vi "信号光谱9-Au-卍 .vi"() -> ()   [LabVIEW 2018]
uses:
  <vilib>/Utility/NIReport.llb/Report Type.ctl
  <vilib>/Utility/file.llb/Write Delimited Spreadsheet (DBL).vi
  <vilib>/Instr/_visa.llb/VISA Configure Serial Port (Instr).vi
  <vilib>/addons/_office/excel.llb/Excel Get Data ([str]).vi
  <vilib>/Utility/NIReport.llb/NI_report.lvclass
  <vilib>/Analysis/NI_AALBase.lvlib
  <vilib>/ptbypt/NI_PtbyPt.lvlib
  <vilib>/Utility/NIReport.llb/NI_ReportGenerationCore.lvlib
  <vilib>/addons/_office/NI_ReportGenerationToolkit.lvlib
  <vilib>/Utility/NIReport.llb/Excel/NI_Excel.lvclass
panel:
  out "temp":i32
  in  "num":i32=2
  in  "角度判断下限":dbl=1.0 format="%#_13g"
  in  "角度判断上限":dbl=4.0 format="%#_13g"
  out "原始峰值":dbl
  out "拟合峰值":dbl
  in  "角度倍乘系数":dbl=1.5
  out "结果展示":dbl[][](array[numeric])=[[37.33100777239877, 2672.955043835526, 29.54153292599307, 222755.0, 50.0], [37.36593979472361, 2672.656498058864, 30.113284142729572, 222833.0, 50.0], [38.96986225690859, 2673.3337152325566, 33.38805102415213, 222910.0, 75.0], [37.39946104045098, 2676.4005085744548, 31.215565446104666, 222948.0, 47.0], [35.862209164247574, 2671.7826876859012, 30.355582265151796, 223028.0, 47.0]]
  out "Δw2>C":bool=TRUE
  out "Δw1>C":bool=TRUE
  out "θi":dbl
  in  "w0":dbl format="%#_13g"
  in  "C=w-w0":dbl=180.0 format="%#_13g"
  in  "上升下降沿/s":dbl format="%.2p"
  in  "延时/s":dbl format="%.2p"
  in  "占空比/%":dbl=3.0 format="%.2p"
  in  "高电平/V":dbl=4.0 format="%.2p"
  in  "频率/Hz":dbl=6000.0 format="%.3p"
  in  "低电平/V":dbl min=0.0 max=5.0 format="%.2p"
  in  "Enable":bool
  in  "上升下降沿":i32(ring)=1 items=["上升沿", "下降沿"]
  in  "输出信号波形":u16(ring) items=["Pulse"]
  out "Output":bool
  in  "VISA 信号发生器":refnum<visa-resource-name>="USB0::0x1AB1::0x0641::DG4E192200870::INSTR"
  out "Output 2":bool
  in  "Enable 2":bool
  in  "上升下降沿/s 2":dbl format="%.2p"
  in  "延时/s 2":dbl format="%.2p"
  in  "占空比/% 2":dbl=3.0 format="%.2p"
  in  "高电平/V 2":dbl=0.002 format="%.2p"
  in  "频率/Hz 2":dbl=6000.0 format="%.3p"
  in  "低电平/V 2":dbl min=0.0 max=5.0 format="%.2p"
  in  "上升下降沿 2":i32(ring)=1 items=["上升沿", "下降沿"]
  in  "输出信号波形 2":u16(ring) items=["Pulse"]
  in  "终止测量":bool
  in  "测量次数":i32=1
  out "best fit":cluster{"Y":dbl[], "Y":dbl[]}[](graph)
  in  "拟合终点":i32=850
  in  "拟合起点":i32=200
  out "angle":dbl
  out "图片地址":string
  in  "开光时间/ms":u32=50
  out "最终存储路径 2":path
  out "照明光error out":errorcluster
  in  "照明光":bool
  in  "stop bits (10: 1 bit)":u16(ring)=10 items=["1.0"=10, "1.5"=15, "2.0"=20]
  in  "parity (0:none)":enum16{"None", "Odd", "Even", "Mark", "Space"}(ring)
  in  "data bits (8)":u16=8 min=5 max=8 step=1
  in  "baud rate":u32=9600 caption="baud rate (115200)" min=9600 max=115200
  in  "照明光VISA":refnum<visa-resource-name>="COM6"
  out "正在测量":bool
  in  "滤波阈值":dbl=3000.0 format="%#_13g"
  out "范围内？":bool[](array[boolean])
  out "w":dbl
  out "xc":dbl
  out "拟合参数":dbl[](array[numeric])
  out "最终存储路径":path
  in  "停止程序":bool
  out "configure error out":errorcluster
  in  "设置参数":bool
  out "output control error  4":errorcluster
  in  "低电平持续输出":bool
  out "output control error  5":errorcluster
  out "output control error":errorcluster
  in  "开始测量":bool
  in  "channel输出口":i32(ring) items=["Channel 1", "Channel 2"]
  out "output control error":errorcluster
  out "Spectrum":cluster{"Y":dbl[], "Y":dbl[]}[](graph)
  out "波长范围":dbl[](array[numeric])
  in  "?":enum32{"IHR 550", "CCD"}(tab)
  in  "Move To\nTarget Positions":bool
  out "Current UniqueID":string="Mono4"
  in  "Mono ID":string(combo)="Mono1"
  in  "Connect":bool
  out "Initialized JY":bool=TRUE
  in  "Force\nInitialization":bool
  in  "Target Grating":string(combo)="2"
  out "Current Description":string="1" caption="Description"
  out "Grating Index":i32=1
  out "Current Grating":dbl=1200.0
  out "Units":string="nm"
  out "Current WL":dbl=897.9988
  out "Exit Mirror\nPosition":i32(ring)=2 items=["EntranceMirror", "ExitMirror", "Front", "Side"]
  out "Entrance Mirror\nPosition":i32(ring)=2 items=["EntranceMirror", "ExitMirror", "Front", "Side"]
  out "Units 2":string="mm"
  out "Front Entrance":dbl
  in  "Target WL":dbl=516.0
  in  "Exit Mirror":u16(ring)=3 caption="Target Position Exit Mirror" items=["Front"=2, "Side"=3]
  in  "Entrance Mirror":u16(ring)=2 caption="Target Position\nEntrance Mirror" items=["Front"=2, "Side"=3]
  in  "Target\nFront Entrance":dbl=2.0
  in  "Commande tab":T1(tab)
  in  "Area Number to Display":i32
  in  "Reformat":bool
  in  "GAIN":u16(ring)=2 caption="Device Name" items=["High Light", "Best Dynamic Range", "High Sensitivity"]
  in  "ADC":u16(ring) caption="Device Name" items=["20 kHz       ", " 1 MHz       ", " 1 MHz Ultra "]
  in  "Number of Areas :":u16=1 min=1 step=1
  in  "Integration time (ms) :":i16=1000
  out "Uniques ID":u16(ring) items=["CCD1", "CCD2"]
  in  "Device Name":u16(ring) items=["Synapse CCD (Lateral)", "Synapse_IGA (Axial)"]
  in  "Signal type :":enum16{"TTL Rising Edge", "TTL Falling Edge"}(ring)=enum."TTL Falling Edge"
  in  "Trigger Type :":u16(ring) items=["On Start"=1, "Per Acquisition"=2]
  in  "trigSigTypeString":string
  in  "trigEventString":string
  in  "Enable InputTriggers :":bool
  in  "Number of Cleans":i32=1
  in  "MultiAcqShutterMode":i32(ring)=3 items=["Open For All Spectra"=1, "Open for Each Spectrum"=3]
  in  "Accumulations:":u16=10 min=1 step=1
  in  "Multi Accumulation mode:":bool
  out "Y Pixels:":i32=256
  out "DataSize":i32=1024
  out "X Pixels:":i32=1024
  out "Firmware\nVersion":string="V1.20 CCD_4000"
  out "initialized ?":bool=TRUE
  in  "Continuous":bool
  in  "CCD Busy":bool
  out "indicator":string="Ready !"
  in  "initialize":bool
  in  "ShutterOpen":bool=TRUE caption="Shutter enable"
  in  "Acquire":bool
  in  "Temperature":bool
  in  "Setup":bool
  out "Acq Time(ms)":u32=3401
  in  "Save Backlight":bool
  in  "cut backlight":bool
  out "backlight":bool=TRUE
  in  "是否拟合":bool
  in  "是否保存":bool
  in  "Close":bool=TRUE
  out "JYCCDLib.IJYCCDReqd":refnum<k7>
  out "areas :":i32[][](array[numeric])=[[1], [1], [1], [1024], [256], [1], [256]]
  in  "Constante de condition\n(Voir l'aide contextuelle)":bool
  out "temp graph":dbl(graph)=-134.538067
  out "ADC Number":i32[](array[numeric])=[0, 1, 2, 3, 4]
  out "Gain Number":i32[](array[numeric])=[10, 11, 12, 13, 8, 2]
  out "trigAddress":i32
  out "Data":i32[][](graph)
  out "error out":errorcluster
  out "Gratings":dbl[](array[numeric])=[1200.0, 300.0]
  out "Backlight":i32[][](graph)
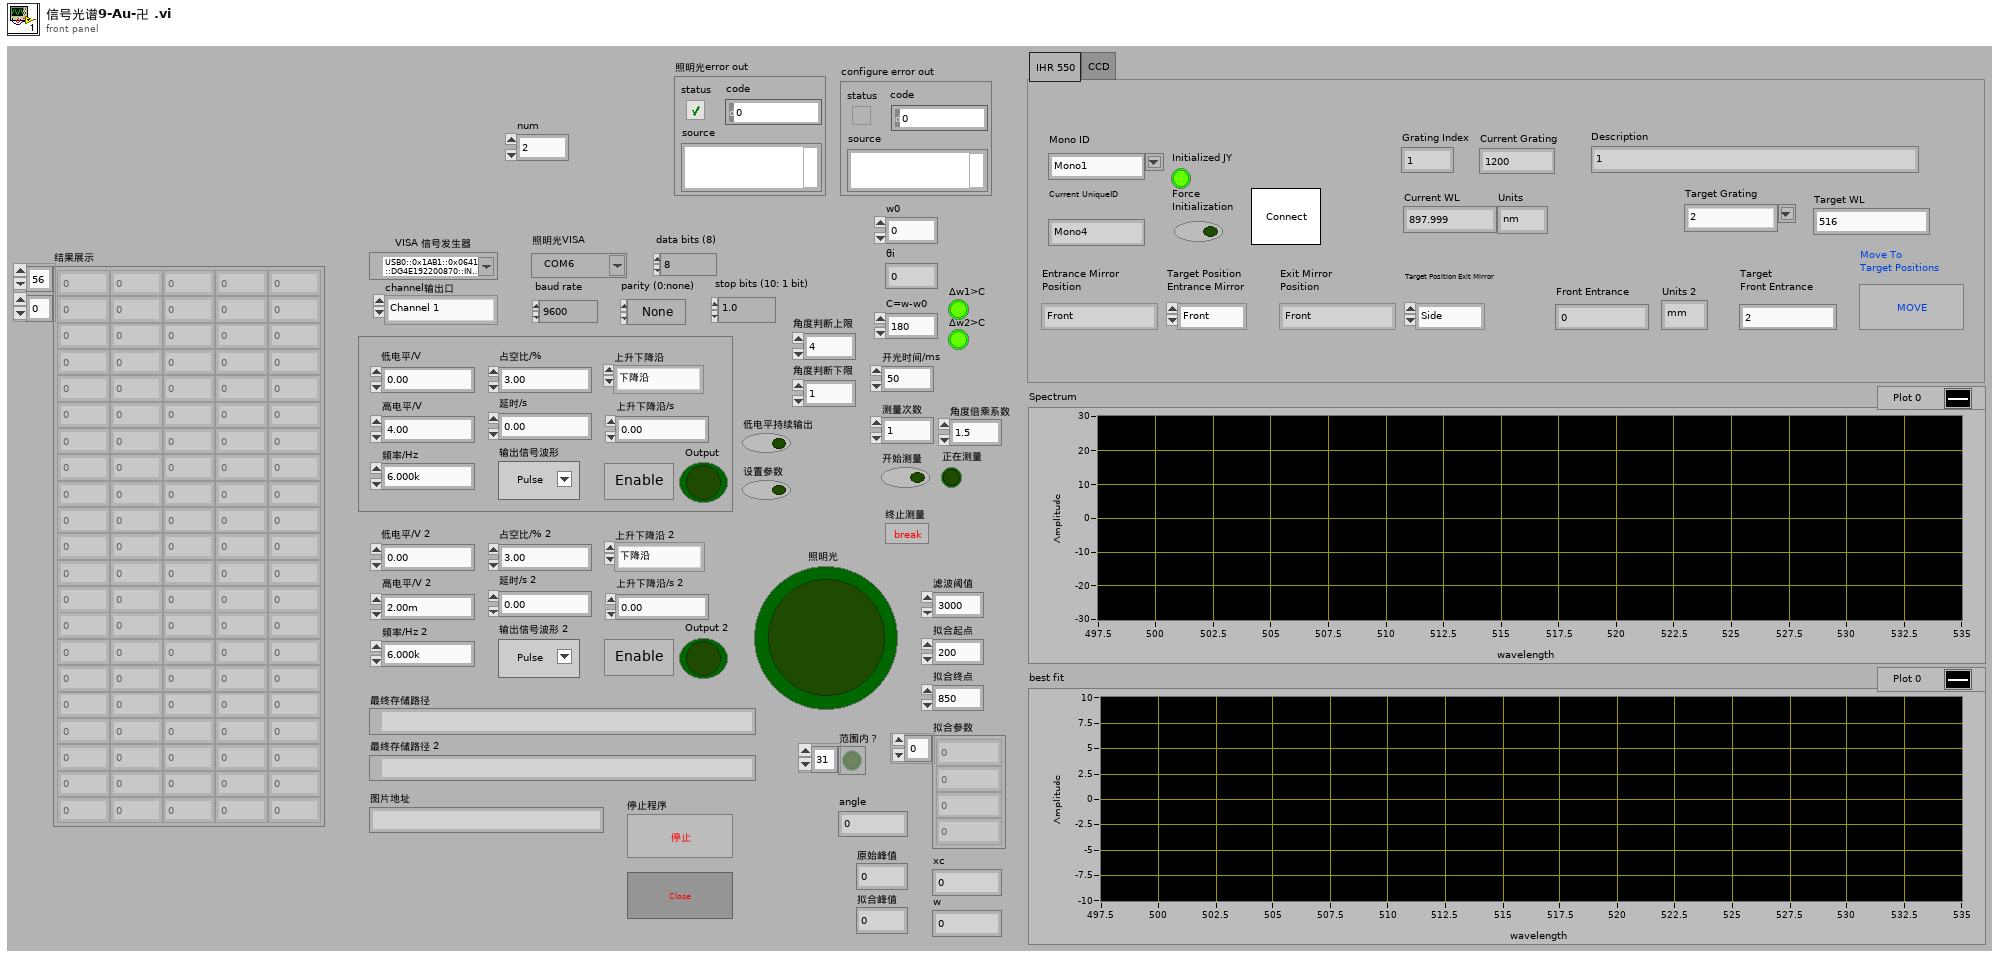
[diagram p1: front panel]
types:
  T1 = enum32{"Settings", "Trigger In", "Multi-Accu.", "Infos"}
  T2 = enum8{"Enabled", "Disabled", "Disabled and Grayed Out"}
  T3 = enum16{"maximized", "minimized", "normal", "no change"}
  T4 = typedef "NI_ReportGenerationCore.lvlib/Report Type.ctl" = enum16{"HTML", "Word", "Excel"}
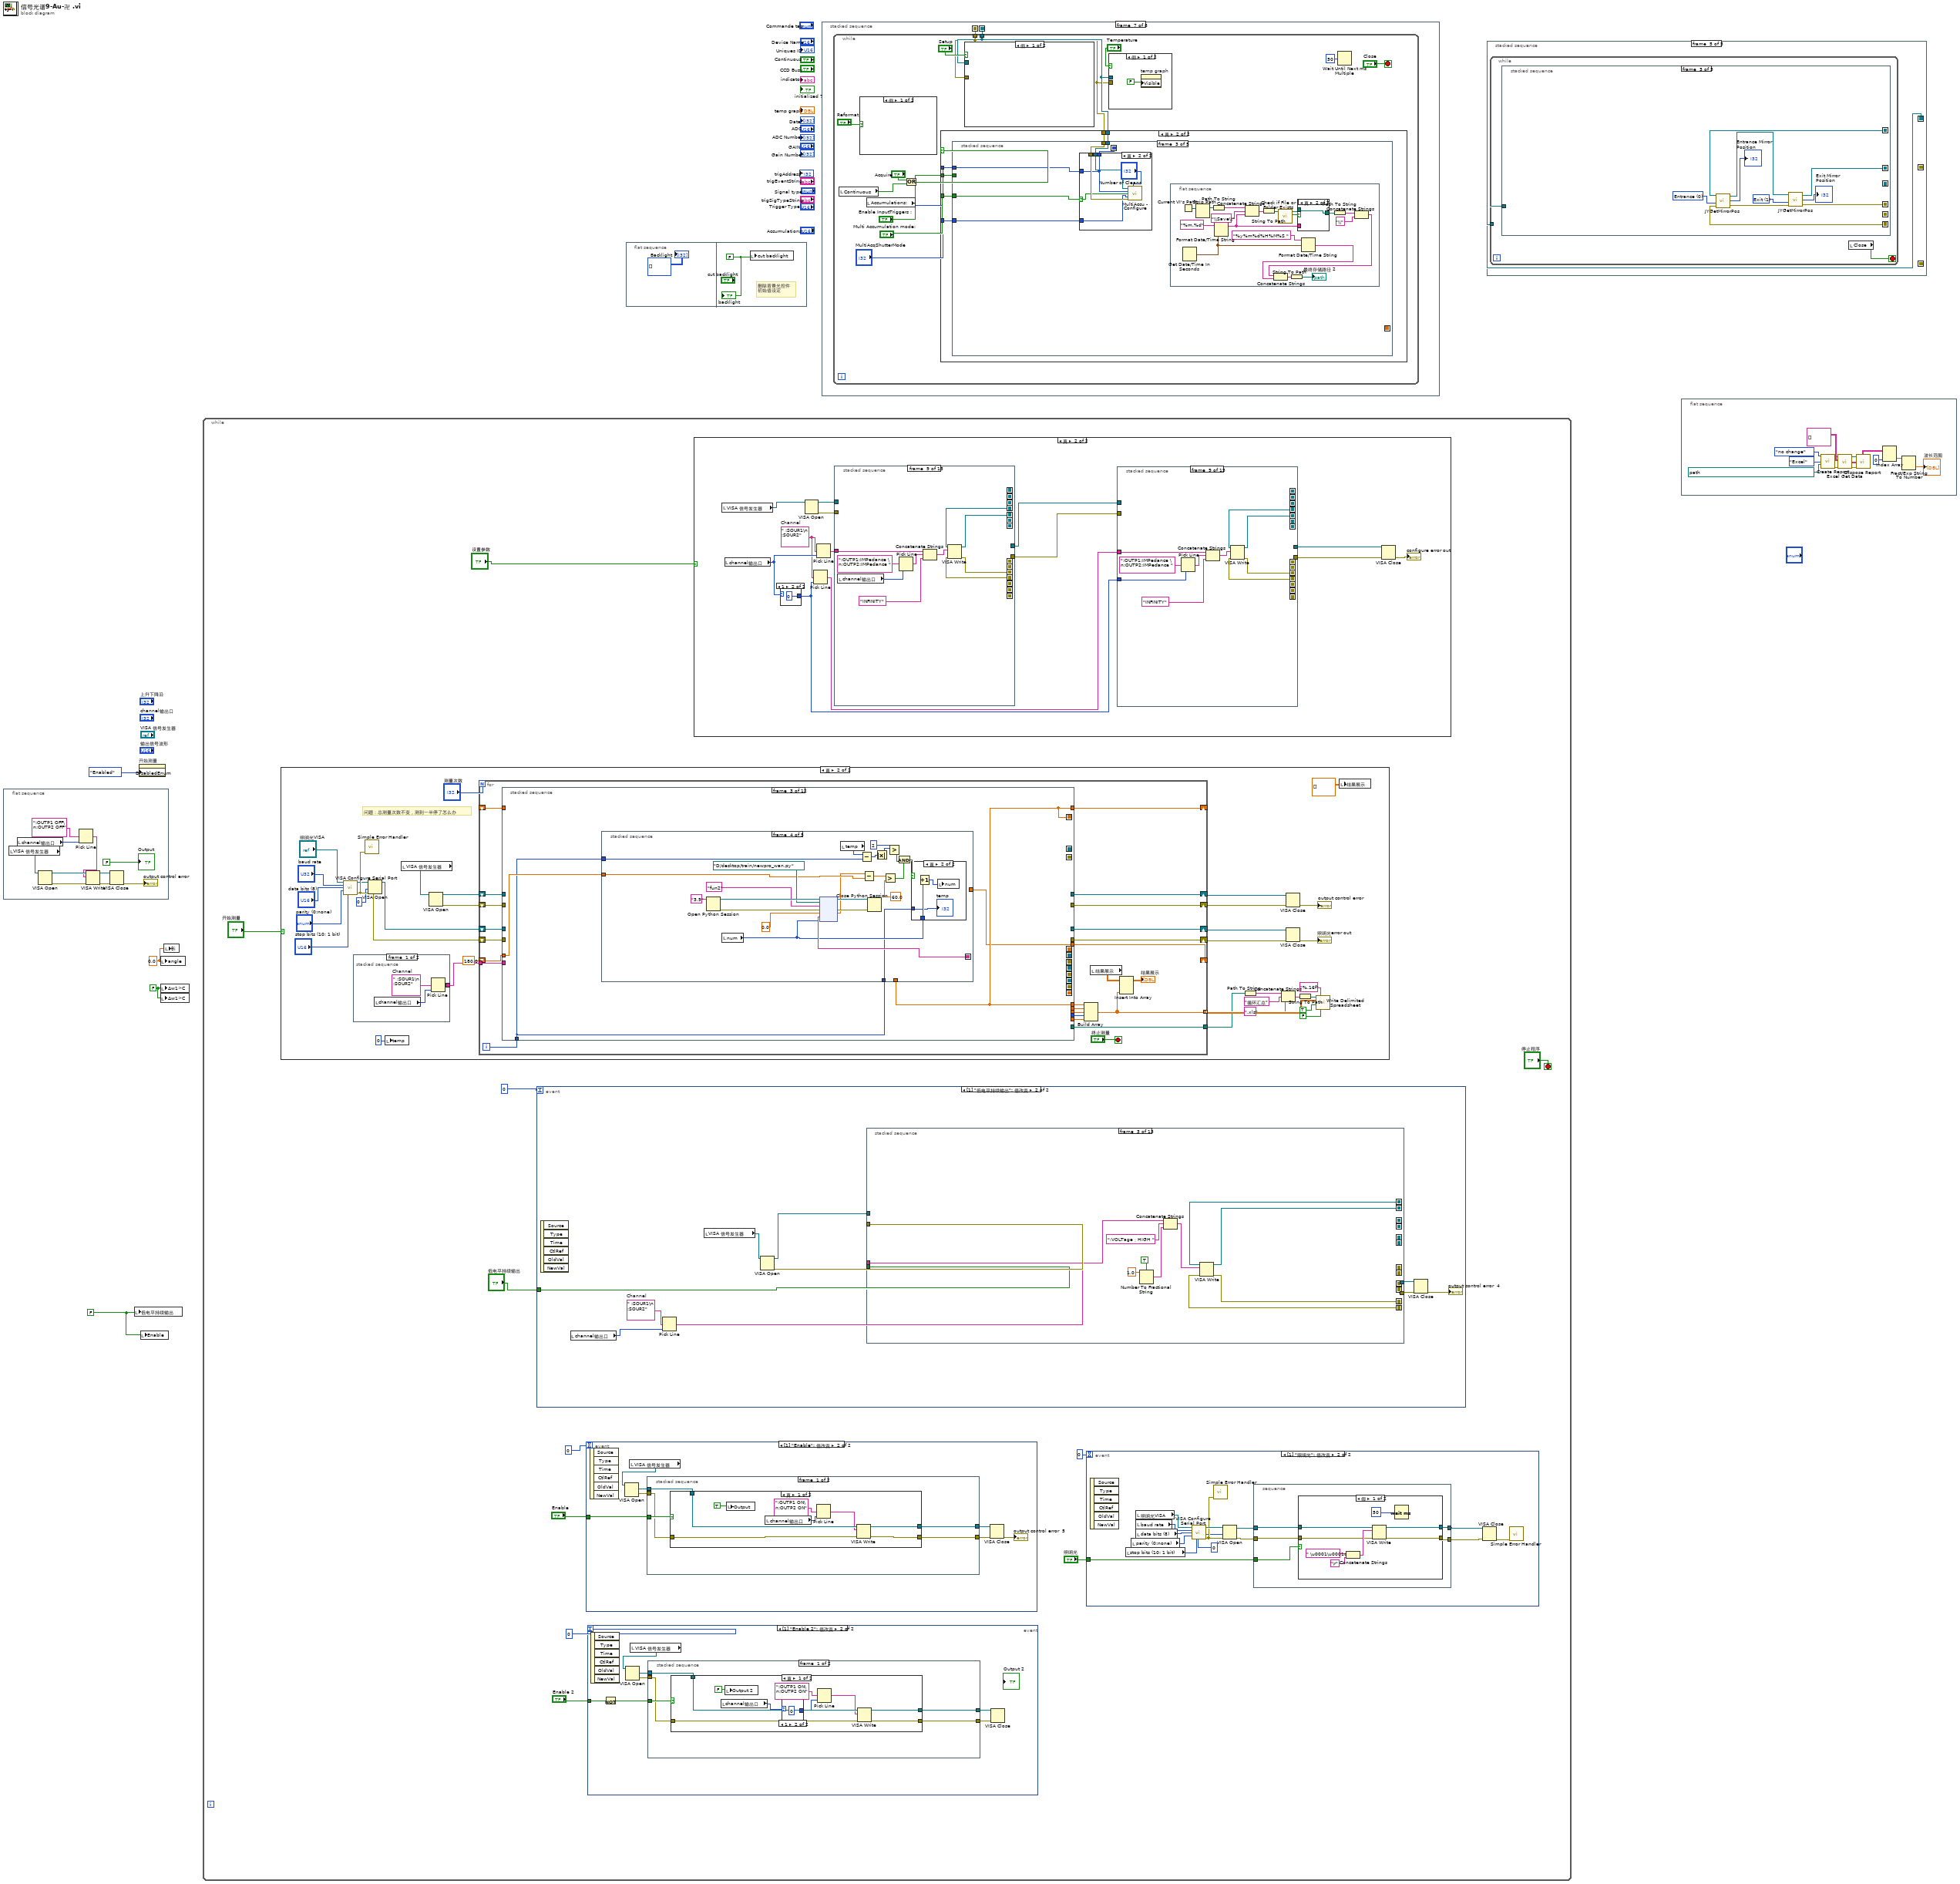
[diagram p0: block diagram]
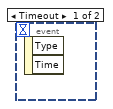
[diagram p2: hidden frame]
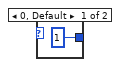
[diagram p3: hidden frame]
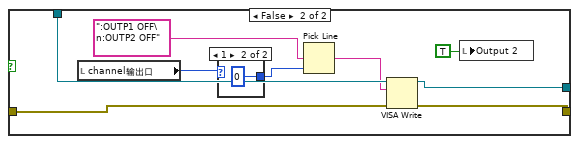
[diagram p4: hidden frame]
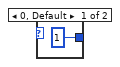
[diagram p5: hidden frame]
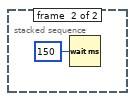
[diagram p6: hidden frame]
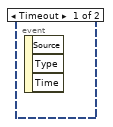
[diagram p7: hidden frame]
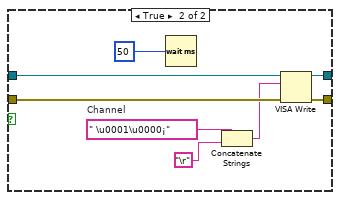
[diagram p8: hidden frame]
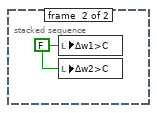
[diagram p10: hidden frame]
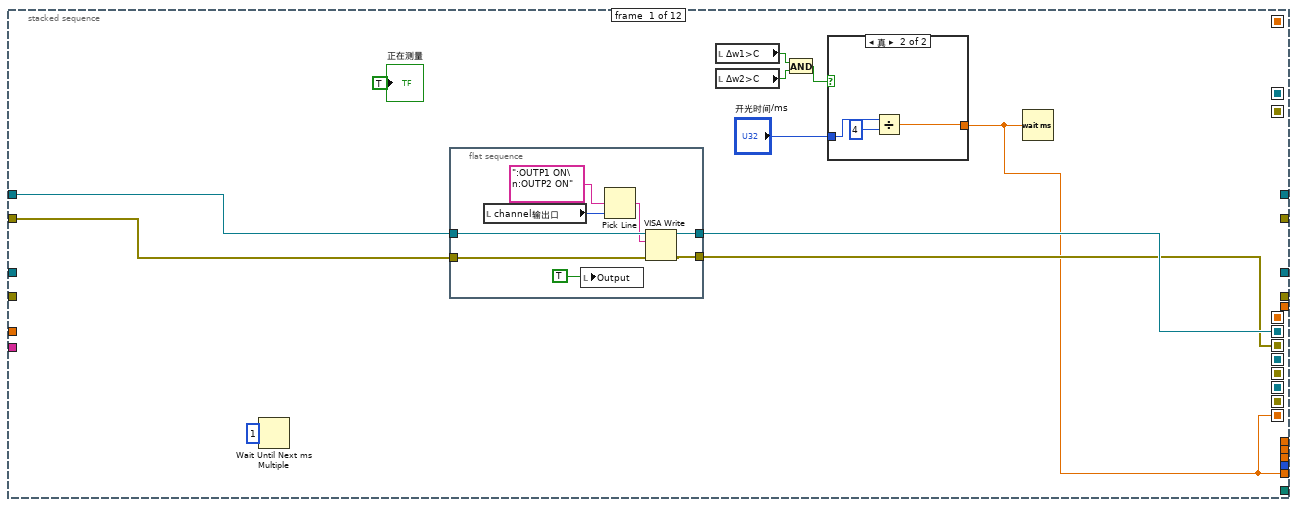
[diagram p11: hidden frame]
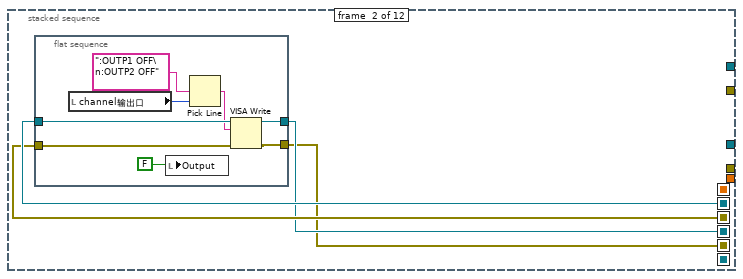
[diagram p13: hidden frame]
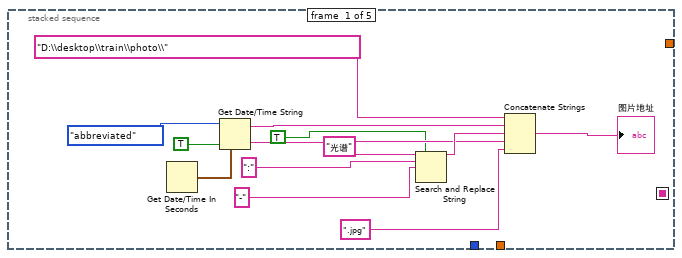
[diagram p14: hidden frame]
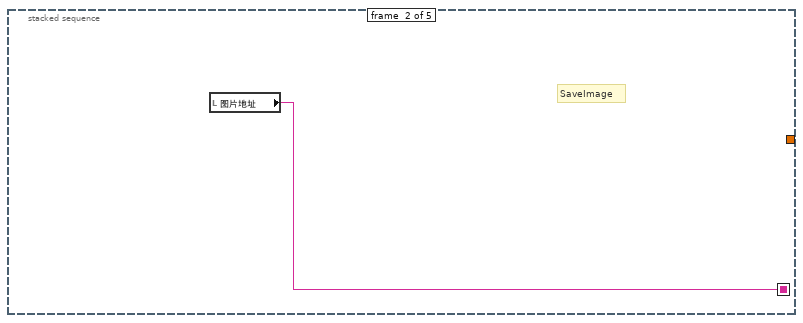
[diagram p15: hidden frame]
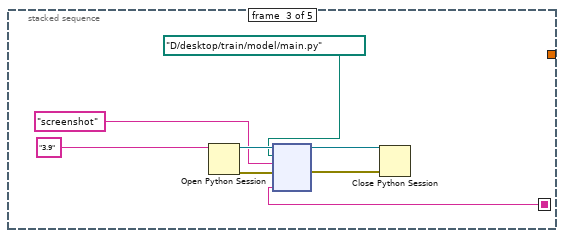
[diagram p16: hidden frame]
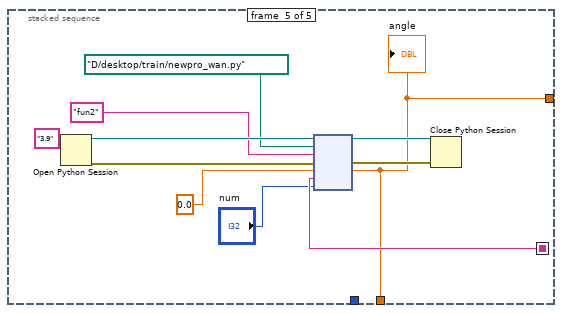
[diagram p18: hidden frame]
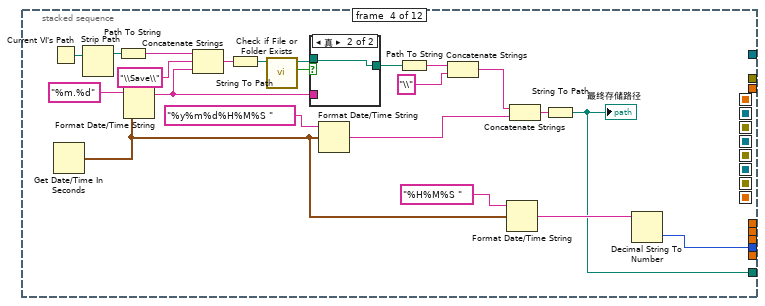
[diagram p19: hidden frame]
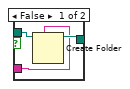
[diagram p20: hidden frame]
diagram:
  w1 = FALSE ("Δw1>C")
  w2 = 0.0 ("angle")
  w3 = FALSE
  n1 = flat-sequence {
    frame #0 {
      n2 = local read "VISA 信号发生器"() -> (w8:refnum<visa-resource-name>)
      n3 = local read "channel输出口"() -> (w6:i32)
      n4 = VISA Open(VISA resource name=w8) -> (VISA resource name=w14:refnum<visa-resource-name>, error out=w13:errorcluster)  [unwired: 4 in]
      n5 = Pick Line(multi-line string=":OUTP1 OFF\n:OUTP2 OFF" ("write buffer"), line index=w6) -> (output string=w5:string)  [unwired: 1 in]
      n6 = VISA Write(VISA resource name=w14, write buffer=w5, error in (no error)=w13) -> (VISA resource name out=w11:refnum<visa-resource-name>, error out=w10:errorcluster)  [unwired: 1 out]
      n7 = VISA Close(VISA resource name=w11, error in (no error)=w10) -> (error out=→"output control error":errorcluster)
      "Output" <- FALSE ("布尔")
    }
  }
  n8 = local write "低电平持续输出"(w3) -> ()
  n9 = property on="开始测量" class="Bool"("DisabledEnum"=T2."Enabled" ("禁用")) -> ()  [unwired: 2 in, 2 out]
  n10 = local write "Enable"(w3) -> ()
  n11 = local write "angle"(w2) -> ()
  n12 = local write "Δw1>C"(w1) -> ()
  n13 = local write "Δw1>C"(w1) -> ()
  n14 = local write "θi"(w2) -> ()
  n15 = while {
    stop <- "停止程序" stop-if-true
    n16 = case shown="真" "开始测量" {
      frame False {
      }
      frame True {
        # "问题：总测量次数不变，测到一半停了怎么办"
        n17 = call-poly "VISA Configure Serial Port"("VISA resource name"="照明光VISA", "baud rate (9600)"="baud rate", "data bits (8)"="data bits (8)", "parity (0:none)"="parity (0:none)", "stop bits (10: 1 bit)"="stop bits (10: 1 bit)") -> ("VISA resource name out"=w120:refnum<visa-resource-name>, "error out"=w121:errorcluster)  [unwired: 9 in]
        n18 = stacked-sequence {
          tunnel: [w130 _] -> w124
          frame #0 {
            w131 = " :SOUR1\n :SOUR2"  # Channel
            n19 = local read "channel输出口"() -> (w132:i32)
            n20 = Pick Line(multi-line string=w131, line index=w132) -> (output string=w130:string)  [unwired: 1 in]
          }
          frame #1 {
            w133 = FALSE ("Δw1>C")
            n21 = local write "Δw1>C"(w133) -> ()
            n22 = local write "Δw2>C"(w133) -> ()
          }
        }
        n23 = call <vilib>:"Simple Error Handler.vi"("error in (no error)"=w121) -> ()  [unwired: 4 in, 5 out]
        n24 = VISA Open(access mode=0, error in (no error)=w121, VISA resource name=w120) -> (VISA resource name=w113:refnum<visa-resource-name>, error out=w112:errorcluster)  [unwired: 2 in]
        n25 = local write "temp"(0 ("temp")) -> ()
        n26 = local read "VISA 信号发生器"() -> (w129:refnum<visa-resource-name>)
        n27 = VISA Open(VISA resource name=w129) -> (VISA resource name=w128:refnum<visa-resource-name>, error out=w127:errorcluster)  [unwired: 4 in]
        n28 = for {
          N: "测量次数" -> [_]
          tunnel: w124 -> [w155]
          shift-right: [w151] -> w123
          shift-left: w128 -> [w157]
          shift-right: [w150] -> w122
          shift-left: w127 -> [w156]
          shift-right: [w149] -> w126
          shift-left: w113 -> [w154]
          shift-right: [w148] -> w125
          shift-left: w112 -> [w153]
          tunnel: [w138] -> w102 mode=indexing
          shift-right: [w143] -> _
          shift-left: _ -> [w142]
          tunnel: [w139] -> w99
          shift-right: [w135] -> _
          shift-left: 180.0 -> [w134]
          i -> [w141]
          stop <- "终止测量" stop-if-true
          n29 = stacked-sequence {
            seq-local: [w164 _ _ _ _ _ _ _ _ _ _ _] -> [_ w184 _ _ _ _ _ _ _ _ _ _]
            seq-local: [w163 _ _ _ _ _ _ _ _ _ _ _] -> [_ w183 _ _ _ _ _ _ _ _ _ _]
            seq-local: [_ _ _ _ _ w299 _ _ _ _ _ _] -> [_ _ _ _ _ _ _ _ w417 _ _ _]
            seq-local: [_ _ _ _ _ w298 _ _ _ _ _ _] -> [_ _ _ _ _ _ _ _ w420 _ _ _]
            seq-local: [_ w182 _ _ _ _ _ _ _ _ _ _] -> [_ _ _ _ w285 _ _ _ _ _ _ _]
            seq-local: [_ w181 _ _ _ _ _ _ _ _ _ _] -> [_ _ _ _ w284 _ _ _ _ _ _ _]
            seq-local: [_ _ _ _ w283 _ _ _ _ _ _ _] -> [_ _ _ _ _ _ _ w403 _ _ _ _]
            seq-local: [_ _ _ _ w282 _ _ _ _ _ _ _] -> [_ _ _ _ _ _ _ w402 _ _ _ _]
            seq-local: [_ _ w196 _ _ _ _ _ _ _ _ _] -> [_ _ _ _ _ _ _ _ _ _ w429 _]
            seq-local: [_ _ _ _ _ _ w312 _ _ _ _ _] -> [_ _ _ _ _ _ _ _ _ _ w424 _]
            seq-local: [w158 _ _ _ _ _ _ _ _ _ _ _] -> [_ _ _ _ _ _ w310 _ _ _ _ _]
            tunnel: w157 -> [w166 _ _ _ _ _ _ _ _ _ _ _]
            tunnel: w156 -> [w165 _ _ _ _ _ _ _ _ _ _ _]
            tunnel: [_ _ _ _ _ _ _ w401 _ _ _ _] -> w151
            tunnel: [_ _ _ _ _ _ _ w400 _ _ _ _] -> w150
            tunnel: w155 -> [_ _ _ _ _ _ _ _ _ _ _ _]
            tunnel: w154 -> [_ _ _ _ _ w302 _ _ _ _ _ _]
            tunnel: w153 -> [_ _ _ _ _ w301 _ _ _ _ _ _]
            tunnel: [_ _ _ _ _ _ _ _ w419 _ _ _] -> w149
            tunnel: [_ _ _ _ _ _ _ _ w418 _ _ _] -> w148
            tunnel: [_ _ w196 _ _ _ _ _ _ _ _ _] -> w147
            tunnel: [_ _ _ _ _ _ w307 _ _ _ _ _] -> w146
            tunnel: [_ _ _ _ _ _ w306 _ _ _ _ _] -> w145
            tunnel: [_ _ _ w257 _ _ _ _ _ _ _ _] -> w144
            tunnel: [w158 _ _ _ _ _ _ _ _ _ _ _] -> w140
            tunnel: [_ _ w196 _ _ _ _ _ _ _ _ _] -> w143
            tunnel: w142 -> [_ _ _ _ _ _ _ _ _ _ w428 _]
            tunnel: w141 -> [_ _ w193 _ _ _ _ _ _ _ w426 _]
            tunnel: [_ _ _ w256 _ _ _ _ _ _ _ _] -> w139
            tunnel: [_ _ w195 _ _ _ _ _ _ _ _ _] -> w135
            tunnel: w134 -> [_ _ w194 _ _ _ _ _ _ _ _ _]
            frame #0 {
              n30 = Wait Until Next ms Multiple(millisecond multiple=u32 1 ("毫秒倍数")) -> ()  [unwired: 1 out]
              n31 = flat-sequence {
                tunnel: w166 -> [w180]
                tunnel: w165 -> [w179]
                tunnel: [w174] -> w164
                tunnel: [w173] -> w163
                frame #0 {
                  n32 = local read "channel输出口"() -> (w176:i32)
                  n33 = local write "Output"(TRUE ("布尔")) -> ()
                  n34 = Pick Line(multi-line string=":OUTP1 ON\n:OUTP2 ON" ("write buffer"), line index=w176) -> (output string=w175:string)  [unwired: 1 in]
                  n35 = VISA Write(VISA resource name=w180, write buffer=w175, error in (no error)=w179) -> (VISA resource name out=w174:refnum<visa-resource-name>, error out=w173:errorcluster)  [unwired: 1 out]
                }
              }
              n36 = local read "Δw1>C"() -> (w160:bool)
              n37 = local read "Δw2>C"() -> (w161:bool)
              n38 = And(x=w160, y=w161) -> (x .and. y?=w159:bool)
              n39 = case shown="真" w159 {
                tunnel: [w169 w170] -> w158
                tunnel: "开光时间/ms" -> [w169 w172]
                frame False {
                }
                frame True {
                  n40 = Divide(x=w172, y=u32 4) -> (x/y=w170:dbl)
                }
              }
              n41 = Wait (ms)(milliseconds to wait=w158) -> ()  [unwired: 1 out]
              "正在测量" <- TRUE
            }
            frame #1 {
              n42 = flat-sequence {
                tunnel: w184 -> [w192]
                tunnel: w183 -> [w191]
                tunnel: [w186] -> w182
                tunnel: [w185] -> w181
                frame #0 {
                  n43 = local read "channel输出口"() -> (w188:i32)
                  n44 = local write "Output"(FALSE ("布尔")) -> ()
                  n45 = Pick Line(multi-line string=":OUTP1 OFF\n:OUTP2 OFF" ("write buffer"), line index=w188) -> (output string=w187:string)  [unwired: 1 in]
                  n46 = VISA Write(VISA resource name=w192, write buffer=w187, error in (no error)=w191) -> (VISA resource name out=w186:refnum<visa-resource-name>, error out=w185:errorcluster)  [unwired: 1 out]
                }
              }
            }
            frame #2 {
              n47 = stacked-sequence {
                seq-local: [_ w210 _ _ _] -> [_ _ w211 w233 w247]
                tunnel: [_ _ _ _ w245] -> w196
                tunnel: [_ _ _ _ w245] -> w195
                tunnel: w194 -> [_ _ _ w229 _]
                tunnel: w193 -> [_ _ _ w225 _]
                tunnel: w193 -> [_ _ _ w223 _]
                frame #0 {
                  n48 = Get Date/Time In Seconds() -> (seconds since 1Jan1904=w206:timestamp)
                  n49 = Get Date/Time String(date format (0)=enum16{"short", "long", "abbreviated"}."abbreviated" ("日期格式(0)"), seconds (now)=w206, want seconds? (F)=TRUE ("需要秒？(F)")) -> (date string=w209:string, time string=w207:string)
                  n50 = Search and Replace String(replace all?=TRUE ("替换全部？(F)"), input string=w207, search string=":" ("搜索字符串"), replace string="-" ("替换字符串(\"\")")) -> (result string=w208:string)  [unwired: 4 in, 3 out]
                  n51 = Concatenate Strings("D:\\desktop\\train\\photo\\", w209, w208, "光谱" ("字符串"), ".jpg" ("字符串")) -> (→"图片地址":string)
                }
                frame #1 {
                  # "SaveImage"
                  n52 = local read "图片地址"() -> (w210:string)
                }
                frame #2 {
                  n53 = Open Python Session(python version="3.9" ("Python version")) -> (session out=w218:refnum<k35>, error out=w216:errorcluster)  [unwired: 2 in]
                  n54 = node(w218, path "D:/desktop/train/model/main.py" ("module path"), "screenshot" ("function name"), w216, w211) -> (w217:refnum<k35>, w215:errorcluster)  [unwired: 3 in, 2 out]
                  n55 = Close Python Session(session in=w217, error in=w215) -> ()  [unwired: 1 out]
                }
                frame #3 {
                  n56 = Open Python Session(python version="3.9" ("Python version")) -> (session out=w240:refnum<k35>, error out=w238:errorcluster)  [unwired: 2 in]
                  n57 = local read "num"() -> (w230:i32)
                  n58 = node(w240, path "D:/desktop/train/newpro_wan.py" ("module path"), "fun2" ("function name"), w238, 0.0, w233, w230) -> (w239:refnum<k35>, w237:errorcluster, w228:dbl)  [unwired: 2 in, 2 out]
                  n59 = local read "temp"() -> (w224:i32)
                  n60 = Subtract(x=w224, y=w223) -> (x-y=w222:i32)
                  n61 = Subtract(x=w228, y=w229) -> (x-y=w232:dbl)
                  n62 = Close Python Session(session in=w239, error in=w237) -> ()  [unwired: 1 out]
                  n63 = Absolute Value(x=w222) -> (abs(x)=w221:i32)
                  n64 = Greater?(x=w232, y=60.0) -> (0:w227:bool)
                  n65 = Greater?(x=w221, y=2) -> (0:w220:bool)
                  n66 = And(x=w227, y=w220) -> (x .and. y?=w226:bool)
                  n67 = case shown="真" w226 {
                    tunnel: w230 -> [_ w244]
                    tunnel: w225 -> [_ w242]
                    frame False {
                    }
                    frame True {
                      n68 = Increment(x=w244) -> (x+1=w243:i32)
                      n69 = local write "num"(w243) -> ()
                      "temp" <- w242
                    }
                  }
                }
                frame #4 {
                  n70 = Open Python Session(python version="3.9" ("Python version")) -> (session out=w254:refnum<k35>, error out=w252:errorcluster)  [unwired: 2 in]
                  n71 = node(w254, path "D:/desktop/train/newpro_wan.py" ("module path"), "fun2" ("function name"), w252, 0.0, w247, "num") -> (w253:refnum<k35>, w251:errorcluster, w245:dbl)  [unwired: 2 in, 2 out]
                  "angle" <- w245
                  n72 = Close Python Session(session in=w253, error in=w251) -> ()  [unwired: 1 out]
                }
              }
            }
            frame #3 {
              n73 = Current VI's Path() -> (path=w266:path)
              n74 = Get Date/Time In Seconds() -> (seconds since 1Jan1904=w259:timestamp)
              n75 = Strip Path(path=w266) -> (stripped path=w267:path)  [unwired: 1 out]
              n76 = Path To String(path=w267) -> (string=w268:string)
              n77 = Format Date/Time String(time format string (%c)="%m.%d" ("时间格式字符串(%c)"), seconds (now)=w259) -> (date/time string=w274:string)  [unwired: 1 in]
              n78 = Concatenate Strings(w268, "\\Save\\" ("字符串"), w274) -> (w269:string)
              n79 = String To Path(string=w269) -> (path=w270:path)
              n80 = call <vilib>:"Check if File or Folder Exists.vi"("path"=w270) -> ("file or folder exists?"=w271:bool, "dup path"=w273:path)  [unwired: 8 in, 1 out]
              n81 = case shown="真" w271 {
                tunnel: [w280 w281] -> w272
                tunnel: w273 -> [w279 w281]
                tunnel: w274 -> [w278 _]
                frame False {
                  n82 = Create Folder(prompt (Create Folder)=w278, path (use dialog)=w279) -> (created path=w280:path)  [unwired: 1 in, 2 out]
                }
                frame True {
                }
              }
              n83 = Format Date/Time String(time format string (%c)="%y%m%d%H%M%S " ("时间格式字符串(%c)"), seconds (now)=w259) -> (date/time string=w277:string)  [unwired: 1 in]
              n84 = Path To String(path=w272) -> (string=w275:string)
              n85 = Concatenate Strings(w275, "\\" ("字符串")) -> (w276:string)
              n86 = Format Date/Time String(time format string (%c)="%H%M%S " ("时间格式字符串(%c)"), seconds (now)=w259) -> (date/time string=w258:string)  [unwired: 1 in]
              n87 = Concatenate Strings(w276, w277) -> (w265:string)
              n88 = String To Path(string=w265) -> (path=w256:path)
              "最终存储路径" <- w256
              n89 = Decimal String To Number(string=w258) -> (number=w257:i32)  [unwired: 2 in, 1 out]
            }
            frame #4 {
              n90 = flat-sequence {
                tunnel: w285 -> [w294]
                tunnel: w284 -> [w293]
                tunnel: [w289] -> w283
                tunnel: [w288] -> w282
                frame #0 {
                  n91 = local read "channel输出口"() -> (w287:i32)
                  n92 = case shown="1" w287 {
                    tunnel: [1 0] -> w286
                    frame 0, Default {
                    }
                    frame 1 {
                    }
                  }
                  n93 = local write "Output 2"(FALSE ("布尔")) -> ()
                  n94 = Pick Line(multi-line string=":OUTP1 OFF\n:OUTP2 OFF" ("write buffer"), line index=w286) -> (output string=w290:string)  [unwired: 1 in]
                  n95 = VISA Write(VISA resource name=w294, write buffer=w290, error in (no error)=w293) -> (VISA resource name out=w289:refnum<visa-resource-name>, error out=w288:errorcluster)  [unwired: 1 out]
                }
              }
            }
            frame #5 {
              w297 = " \u0001\u0001¢"  # Channel
              n96 = Wait (ms)(milliseconds to wait=1200) -> ()  [unwired: 1 out]
              n97 = Concatenate Strings(w297, "\r") -> (w303:string)
              n98 = local write "照明光"(FALSE ("照明光")) -> ()
              n99 = VISA Write(VISA resource name=w302, write buffer=w303, error in (no error)=w301) -> (VISA resource name out=w299:refnum<visa-resource-name>, error out=w298:errorcluster)  [unwired: 1 out]
            }
            frame #6 {
              n100 = local read "Area Number to Display"() -> (w353:i32)
              n101 = local read "JYCCDLib.IJYCCDReqd"() -> (w349:refnum<k7>)
              n102 = Get Date/Time In Seconds() -> (seconds since 1Jan1904=w362:timestamp)
              n103 = local read "最终存储路径"() -> (w376:path)
              n104 = Get Date/Time String(date format (0)=enum16{"short", "long", "abbreviated"}."abbreviated" ("日期格式(0)"), seconds (now)=w362, want seconds? (F)=TRUE ("需要秒？(F)")) -> (date string=w370:string, time string=w365:string)
              n105 = call "MultiAccu - Acquire spectral.vi"("error in"=errorcluster {"status"=FALSE, "code"=0, "source"=""}, "Accumulations:"=u16 1, "ShutterOpen"=TRUE, "JYCCDLib.IJYCCDReqd"=w349) -> ("Acq Time(ms)"=w355:u32, "Array Out"=w354:i32[][][])  [unwired: 1 out]
              n106 = local write "Acq Time(ms)"(w355) -> ()
              n107 = local read "cut backlight"() -> (w337:bool)
              n108 = local read "backlight"() -> (w335:bool)
              n109 = Search and Replace String(replace all?=TRUE ("替换全部？(F)"), input string=w365, search string=":" ("搜索字符串"), replace string="-" ("替换字符串(\"\")")) -> (result string=w369:string)  [unwired: 4 in, 3 out]
              n110 = Path To String(path=w376) -> (string=w359:string)
              n111 = And(x=w337, y=w335) -> (x .and. y?=w336:bool)
              n112 = call "Array reset dimension.vi"("Area Number"=w353, "Array In"=w354) -> ("Array Out"=w339:i32[][])
              n113 = Concatenate Strings(w359, w370, w369, "光谱" ("字符串"), ".xls" ("字符串")) -> (w374:string)
              n114 = case shown="真" w336 {
                tunnel: [w396 w398] -> w338
                tunnel: w339 -> [w396 w397]
                frame False {
                }
                frame True {
                  n115 = local read "Backlight"() -> (w399:i32[][])
                  n116 = Subtract(x=w397, y=w399) -> (x-y=w398:i32[][])
                }
              }
              n117 = String To Path(string=w374) -> (path=w375:path)
              n118 = local write "Data"(w339) -> ()
              n119 = local read "波长范围"() -> (w318:dbl[])
              n120 = Index Array(array=w338, index (row)=0 ("索引 (行)")) -> (element=w377:i32[])  [unwired: 1 in]
              n121 = Reverse 1D Array(array=w377) -> (reversed array=w315:i32[])
              n122 = local read "angle"() -> (w317:dbl)
              n123 = local read "拟合起点"() -> (w325:i32)
              n124 = local read "拟合终点"() -> (w327:i32)
              n125 = call <vilib>:"Median Filter.vi"("left rank"=6, "X"=w315) -> ("Filtered X"=w314:dbl[])  [unwired: 8 in, 1 out]
              n126 = Build Array(w317, w310, 0.0 ("元素")) -> (w316:dbl[])
              n127 = Subtract(x=w327, y=w325) -> (x-y=w324:i32)
              n128 = call "Convert to Dynamic Data"("Array"=w318) -> ("Dynamic Data Type"=w346:dynamicdata)  [unwired: 3 in]
              n129 = call "Convert to Dynamic Data2"("Array"=w315) -> ("Dynamic Data Type"=w345:dynamicdata)  [unwired: 3 in]
              n130 = Array Subset(array=w318, index=w325, length=w324) -> (w323:dbl[])
              n131 = call "Build XY Graph"("Y Input"=w345, "X Input"=w346) -> ("XY Graph"=→"Spectrum":cluster{"Y":dbl[], "Y":dbl[]}[])  [unwired: 8 in, 1 out]
              n132 = call "转换至动态数据4"("Array"=w323) -> ("Dynamic Data Type"=w343:dynamicdata)  [unwired: 3 in]
              n133 = In Range and Coerce(upper limit="滤波阈值", x=w314, lower limit=-100.0) -> (In Range?=w330:bool[])  [unwired: 1 out]
              "范围内？" <- w330
              n134 = Not(x=w330) -> (.not. x?=w329:bool[])
              n135 = Or Array Elements(Boolean array=w329) -> (logical OR=w332:bool)
              n136 = local read "X Pixels:"() -> (w331:i32)
              n137 = local read "波长范围"() -> (w319:dbl[])
              n138 = local read "滤波阈值"() -> (w328:dbl)
              n139 = case shown="真" w332 {
                tunnel: w331 -> [_ w383]
                tunnel: w314 -> [w379 w382]
                tunnel: [w379 w381] -> w308
                tunnel: w328 -> [_ w380]
                frame False {
                }
                frame True {
                  n140 = for {
                    N: w383 -> [_]
                    tunnel: w382 -> [w387] mode=indexing
                    tunnel: [w386] -> w381 mode=indexing
                    shift-right: [w386] -> _
                    shift-left: _ -> [w385]
                    tunnel: w380 -> [w384]
                    n141 = Greater?(x=w387, y=w384) -> (0:w389:bool)
                    n142 = Less?(x=w387, y=-100.0) -> (x < y?=w390:bool)
                    n143 = Or(x=w389, y=w390) -> (x .or. y?=w388:bool)
                    n144 = case shown="真" w388 {
                      tunnel: w387 -> [w392 _]
                      tunnel: [w392 w394] -> w386
                      tunnel: w385 -> [_ w395]
                      frame False {
                      }
                      frame True {
                        n145 = call <vilib>:"Median Filter PtByPt.vi"("rank"=5, "x"=w395) -> ("Filtered x"=w394:dbl)  [unwired: 2 in, 1 out]
                      }
                    }
                  }
                }
              }
              n146 = Array Subset(array=w308, index=w325, length=w324) -> (w326:dbl[])
              n147 = call "转换至动态数据3"("Array"=w326) -> ("Dynamic Data Type"=w344:dynamicdata)  [unwired: 3 in]
              n148 = call "曲线拟合"("Locations"=w343, "Signals"=w344) -> ("best fit"=w348:dynamicdata, "non-linear coefficients"=w347:dynamicdata)  [unwired: 5 in, 3 out]
              n149 = call "从动态数据转换"("Dynamic Data Type"=w347) -> ("Array"=w340:dbl[])  [unwired: 3 in]
              "拟合参数" <- w340
              n150 = call "从动态数据转换2"("Dynamic Data Type"=w348) -> ("Array"=w309:dbl[])  [unwired: 3 in]
              n151 = Build Array(w318, w314, w309, w340, w316) -> (w378:dbl[][])
              n152 = call-poly <vilib>:"Write Delimited Spreadsheet.vi"("file path (dialog if empty)"=w375, "format (%.3f)"="%.16f", "2D data"=w378, "append to file? (new file:F)"=TRUE ("append to file? (F)"), "transpose? (no:F)"=TRUE ("transpose? (F)")) -> ()  [unwired: 9 in, 2 out]
              n153 = Index Array(array=w340, index #1=0 ("索引"), index #2=1 ("索引")) -> (element #1=→"xc":dbl, element #2=w312:dbl)
              "w" <- w312
              n154 = Bundle("波长范围"=w319, "Filtered X"=w308) -> (w322:cluster{"波长范围 ":dbl[], "Filtered X":dbl[]})  [unwired: 1 in]
              n155 = Bundle(w323, "Array"=w309) -> (w321:cluster{dbl[], "Array":dbl[]})  [unwired: 1 in]
              n156 = Array Max & Min(array=w309) -> (max value=w306:dbl)  [unwired: 3 out]
              "拟合峰值" <- w306
              n157 = Array Max & Min(array=w308) -> (max value=w307:dbl)  [unwired: 3 out]
              "原始峰值" <- w307
              n158 = Build Array(w322, w321) -> (w320:cluster{"波长范围 ":dbl[], "Array":dbl[]}[])
              n159 = local write "best fit"(w320) -> ()
            }
            frame #7 {
              n160 = flat-sequence {
                tunnel: w403 -> [w412]
                tunnel: w402 -> [w411]
                tunnel: [w407] -> w401
                tunnel: [w406] -> w400
                frame #0 {
                  n161 = local read "channel输出口"() -> (w405:i32)
                  n162 = case shown="1" w405 {
                    tunnel: [1 0] -> w404
                    frame 0, Default {
                    }
                    frame 1 {
                    }
                  }
                  n163 = local write "Output 2"(TRUE ("布尔")) -> ()
                  n164 = Pick Line(multi-line string=":OUTP1 ON\n:OUTP2 ON" ("write buffer"), line index=w404) -> (output string=w408:string)  [unwired: 1 in]
                  n165 = VISA Write(VISA resource name=w412, write buffer=w408, error in (no error)=w411) -> (VISA resource name out=w407:refnum<visa-resource-name>, error out=w406:errorcluster)  [unwired: 1 out]
                }
              }
            }
            frame #8 {
              w415 = " \u0001\u0000¡"  # Channel
              n166 = Concatenate Strings(w415, "\r") -> (w421:string)
              n167 = VISA Write(VISA resource name=w417, write buffer=w421, error in (no error)=w420) -> (VISA resource name out=w419:refnum<visa-resource-name>, error out=w418:errorcluster)  [unwired: 1 out]
              n168 = local write "照明光"(TRUE ("照明光")) -> ()
            }
            frame #9 {
              n169 = Wait (ms)(milliseconds to wait=1200) -> ()  [unwired: 1 out]
            }
            frame #10 {
              n170 = Greater Or Equal?(x=w426, y=1) -> (x >= y?=w427:bool)
              n171 = case shown="真" w427 {
                tunnel: w429 -> [_ w435]
                tunnel: w428 -> [_ w436]
                tunnel: w424 -> [w430 w437]
                frame False {
                  n172 = local write "w0"(w430) -> ()
                }
                frame True {
                  n173 = local read "Δw1>C"() -> (w434:bool)
                  n174 = case shown="真" w434 {
                    tunnel: w437 -> [w456 w476]
                    tunnel: w436 -> [w446 _]
                    tunnel: w435 -> [w447 _]
                    frame False {
                      # "判断Δw突变位置并记录当前θ值"
                      # "根据θ变化速度改变开光时间"
                      n175 = local read "w0"() -> (w454:dbl)
                      n176 = Subtract(x=w447, y=w446) -> (x-y=w449:dbl)
                      n177 = local read "开光时间/ms"() -> (w452:u32)
                      n178 = Subtract(x=w454, y=w456) -> (x-y=w459:dbl)
                      n179 = Absolute Value(x=w449) -> (abs(x)=w451:dbl)
                      n180 = Absolute Value(x=w459) -> (abs(x)=w457:dbl)
                      n181 = Greater Or Equal?(x=w451, y="角度判断上限") -> (x >= y?=w450:bool)
                      n182 = Greater Or Equal?(x=w457, y="C=w-w0") -> (x >= y?=w455:bool)
                      n183 = case shown="真" w455 {
                        tunnel: w446 -> [_ w474]
                        frame False {
                          w472 = FALSE ("Δw1>C")
                          n184 = local write "Δw1>C"(w472) -> ()
                          n185 = local write "Δw2>C"(w472) -> ()
                        }
                        frame True {
                          "θi" <- w474
                          "Δw1>C" <- TRUE ("布尔")
                        }
                      }
                      n186 = case shown="假" w450 {
                        tunnel: w451 -> [w464 _]
                        tunnel: w452 -> [w461 w471]
                        tunnel: [w460 w469] -> w453
                        frame False {
                          n187 = Less Or Equal?(x=w464, y="角度判断下限") -> (x <= y?=w462:bool)
                          n188 = case shown="真" w462 {
                            tunnel: w461 -> [w465 w468]
                            tunnel: [w465 w467] -> w460
                            frame False {
                            }
                            frame True {
                              n189 = Multiply(x=w468, y="角度倍乘系数") -> (x*y=w467:dbl)
                            }
                          }
                        }
                        frame True {
                          n190 = Divide(x=w471, y=1.6) -> (x/y=w469:dbl)
                        }
                      }
                      n191 = local write "开光时间/ms"(w453) -> ()
                    }
                    frame True {
                      # "再次判断Δw，排除坏点影响"
                      n192 = local read "Δw2>C"() -> (w475:bool)
                      n193 = case shown="假" w475 {
                        tunnel: w476 -> [w481 _]
                        frame False {
                          n194 = local read "C=w-w0"() -> (w478:dbl)
                          n195 = local read "w0"() -> (w482:dbl)
                          n196 = Subtract(x=w482, y=w481) -> (x-y=w484:dbl)
                          n197 = Absolute Value(x=w484) -> (abs(x)=w483:dbl)
                          n198 = Add(x=w478, y=0) -> (x+y=w477:dbl)
                          n199 = Greater Or Equal?(x=w483, y=w477) -> (x >= y?=w480:bool)
                          n200 = case shown="真" w480 {
                            frame False {
                              n201 = local write "θi"(0.0 ("θi")) -> ()
                              n202 = local write "Δw1>C"(FALSE ("Δw1>C")) -> ()
                            }
                            frame True {
                              "Δw2>C" <- TRUE
                            }
                          }
                        }
                        frame True {
                        }
                      }
                    }
                  }
                  n203 = local read "Δw1>C"() -> (w432:bool)
                  n204 = local read "Δw2>C"() -> (w433:bool)
                  n205 = And(x=w432, y=w433) -> (x .and. y?=w431:bool)
                  n206 = case shown="假" w431 {
                    tunnel: w435 -> [_ w438]
                    frame False {
                    }
                    frame True {
                      # "4°后重置指示灯状态"
                      n207 = local read "θi"() -> (w442:dbl)
                      n208 = Subtract(x=w438, y=w442) -> (x-y=w443:dbl)
                      n209 = Absolute Value(x=w443) -> (abs(x)=w441:dbl)
                      n210 = Greater?(x=w441, y=4.0) -> (0:w439:bool)
                      n211 = case shown="真" w439 {
                        frame False {
                        }
                        frame True {
                          w444 = FALSE ("Δw1>C")
                          n212 = local write "Δw1>C"(w444) -> ()
                          n213 = local write "Δw2>C"(w444) -> ()
                          n214 = local write "θi"(0.0 ("θ")) -> ()
                        }
                      }
                    }
                  }
                }
              }
            }
            frame #11 {
              n215 = local write "正在测量"(FALSE) -> ()
            }
          }
          n216 = Build Array(w147, w146, w145, w144, w140) -> (w138:dbl[])
          n217 = local read "结果展示"() -> (w137:dbl[][])
          n218 = Insert Into Array(array=w137, new element=w138) -> (→"结果展示":dbl[][])  [unwired: 2 in]
        }
        n219 = Path To String(path=w99) -> (string=w108:string)
        n220 = Concatenate Strings(w108, "循环汇总" ("字符串"), ".xls" ("字符串")) -> (w107:string)
        n221 = VISA Close(VISA resource name=w123, error in (no error)=w122) -> (error out=→"output control error":errorcluster)
        n222 = VISA Close(VISA resource name=w126, error in (no error)=w125) -> (error out=→"照明光error out":errorcluster)
        n223 = String To Path(string=w107) -> (path=w106:path)
        n224 = call-poly <vilib>:"Write Delimited Spreadsheet.vi"("file path (dialog if empty)"=w106, "format (%.3f)"="%.16f", "2D data"=w102, "append to file? (new file:F)"=TRUE ("append to file? (F)"), "transpose? (no:F)"=FALSE ("transpose? (F)")) -> ()  [unwired: 9 in, 2 out]
        n225 = local write "结果展示"(dbl[][] [] ("结果展示")) -> ()
      }
    }
    n226 = event shown="[1] \"低电平持续输出\": 值改变" {
      selector: _ -> [_ _]
      dyn-events: _ -> [_ _]
      timeout: u32 0 ("Time") -> [_ _]
      tunnel: "低电平持续输出" -> [_ w518]
      event Timeout {
        n227 = event-data() -> ()  [unwired: 1 in, 2 out]
      }
      event "低电平持续输出": Value Change {
        w522 = " :SOUR1\n :SOUR2"  # Channel
        n228 = event-data() -> ()  [unwired: 1 in, 6 out]
        n229 = local read "channel输出口"() -> (w523:i32)
        n230 = Pick Line(multi-line string=w522, line index=w523) -> (output string=w521:string)  [unwired: 1 in]
        n231 = local read "VISA 信号发生器"() -> (w526:refnum<visa-resource-name>)
        n232 = VISA Open(VISA resource name=w526) -> (VISA resource name=w525:refnum<visa-resource-name>, error out=w524:errorcluster)  [unwired: 4 in]
        n233 = stacked-sequence {
          seq-local: [w532 _ _ _ _ _ _ _ _ _ _ _ _] -> [_ _ w547 _ _ _ _ _ _ _ _ _ _]
          seq-local: [w531 _ _ _ _ _ _ _ _ _ _ _ _] -> [_ _ w546 _ _ _ _ _ _ _ _ _ _]
          seq-local: [_ _ w545 _ _ _ _ _ _ _ _ _ _] -> [_ _ _ _ w550 _ _ _ _ _ _ _ _]
          seq-local: [_ _ w544 _ _ _ _ _ _ _ _ _ _] -> [_ _ _ _ w551 _ _ _ _ _ _ _ _]
          seq-local: [_ _ _ _ w559 _ _ _ _ _ _ _ _] -> [_ _ _ _ _ _ w570 _ _ _ _ _ _]
          seq-local: [_ _ _ _ w558 _ _ _ _ _ _ _ _] -> [_ _ _ _ _ _ w569 _ _ _ _ _ _]
          seq-local: [_ _ _ _ _ _ w563 _ _ _ _ _ _] -> [_ _ _ _ _ _ _ _ w573 _ _ _ _]
          seq-local: [_ _ _ _ _ _ w562 _ _ _ _ _ _] -> [_ _ _ _ _ _ _ _ w572 _ _ _ _]
          seq-local: [_ _ _ _ _ _ _ _ w576 _ _ _ _] -> [_ _ _ _ _ _ _ _ _ _ w587 _ _]
          seq-local: [_ _ _ _ _ _ _ _ w575 _ _ _ _] -> [_ _ _ _ _ _ _ _ _ _ w586 _ _]
          seq-local: [_ _ _ _ _ _ _ _ _ _ w584 _ _] -> [_ _ _ _ _ _ _ _ _ _ _ _ w601]
          seq-local: [_ _ _ _ _ _ _ _ _ _ w583 _ _] -> [_ _ _ _ _ _ _ _ _ _ _ _ w600]
          tunnel: w525 -> [w537 _ _ _ _ _ _ _ _ _ _ _ _]
          tunnel: w524 -> [w530 _ _ _ _ _ _ _ _ _ _ _ _]
          tunnel: w521 -> [w529 _ w543 _ w556 _ w567 _ w577 _ w590 _ _]
          tunnel: [_ _ _ _ _ _ _ _ _ _ _ _ w599] -> w520
          tunnel: [_ _ _ _ _ _ _ _ _ _ _ _ w597] -> w519
          tunnel: w518 -> [_ _ _ _ _ _ _ _ _ _ _ _ w598]
          frame #0 {
            w534 = " PULSe"  # Function Command
            n234 = local read "输出信号波形"() -> (w528:u16)
            n235 = Concatenate Strings(w529, ":FUNC" ("string (\"\")")) -> (w535:string)
            n236 = Pick Line(string ("")=w535, multi-line string=w534, line index=w528) -> (output string=w533:string)
            n237 = VISA Write(VISA resource name=w537, write buffer=w533, error in (no error)=w530) -> (VISA resource name out=w532:refnum<visa-resource-name>, error out=w531:errorcluster)  [unwired: 1 out]
          }
          frame #1 {
            n238 = Wait (ms)(milliseconds to wait=u32 150) -> ()  [unwired: 1 out]
          }
          frame #2 {
            n239 = Number To Fractional String(use system decimal point (T)=TRUE ("使用系统小数点(T)"), number=1.0 ("数字")) -> (F-format string=w541:string)  [unwired: 2 in]
            n240 = Concatenate Strings ("连接字符串")(w543, ":VOLTage：HIGH ", w541) -> (w540:string)
            n241 = VISA Write(VISA resource name=w547, write buffer=w540, error in (no error)=w546) -> (VISA resource name out=w545:refnum<visa-resource-name>, error out=w544:errorcluster)  [unwired: 1 out]
          }
          frame #3 {
            n242 = Wait (ms)(milliseconds to wait=u32 150) -> ()  [unwired: 1 out]
          }
          frame #4 {
            # "1 电压偏置"
            n243 = Number To Fractional String(use system decimal point (T)=TRUE ("使用系统小数点(T)"), number=0.0 ("数字")) -> (F-format string=w554:string)  [unwired: 2 in]
            n244 = Concatenate Strings(w556, ":VOLTage:LOW ", w554) -> (w555:string)
            n245 = VISA Write(VISA resource name=w550, write buffer=w555, error in (no error)=w551) -> (VISA resource name out=w559:refnum<visa-resource-name>, error out=w558:errorcluster)  [unwired: 1 out]
          }
          frame #5 {
            n246 = Wait (ms)(milliseconds to wait=u32 150) -> ()  [unwired: 1 out]
          }
          frame #6 {
            n247 = local read "channel输出口"() -> (w565:i32)
            n248 = Pick Line(multi-line string=":OUTP1:IMPedance \n:OUTP2:IMPedance " ("write buffer"), line index=w565) -> (output string=w564:string)  [unwired: 1 in]
            n249 = Concatenate Strings ("连接字符串")(w567, w564, "INFINITY") -> (w568:string)
            n250 = VISA Write(VISA resource name=w570, write buffer=w568, error in (no error)=w569) -> (VISA resource name out=w563:refnum<visa-resource-name>, error out=w562:errorcluster)  [unwired: 1 out]
          }
          frame #7 {
            n251 = Wait (ms)(milliseconds to wait=u32 150) -> ()  [unwired: 1 out]
          }
          frame #8 {
            n252 = Number To Fractional String(use system decimal point (T)=TRUE ("使用系统小数点(T)"), number=0.0 ("数字")) -> (F-format string=w580:string)  [unwired: 2 in]
            n253 = Concatenate Strings(w577, ":PULSe:DELay ", w580) -> (w578:string)
            n254 = VISA Write(VISA resource name=w573, write buffer=w578, error in (no error)=w572) -> (VISA resource name out=w576:refnum<visa-resource-name>, error out=w575:errorcluster)  [unwired: 1 out]
          }
          frame #9 {
            n255 = Wait (ms)(milliseconds to wait=u32 150) -> ()  [unwired: 1 out]
          }
          frame #10 {
            w591 = ":LEADing\n:TRAiling "  # Channel
            w595 = ":PULSe:TRANsition"  # VOLTage:Offset
            n256 = local read "上升下降沿"() -> (w592:i32)
            n257 = Pick Line(multi-line string=w591, line index=w592) -> (output string=w588:string)  [unwired: 1 in]
            n258 = Number To Fractional String(use system decimal point (T)=TRUE ("使用系统小数点(T)"), number=0.0 ("数字")) -> (F-format string=w589:string)  [unwired: 2 in]
            n259 = Concatenate Strings(w590, w595, w588, w589) -> (w593:string)
            n260 = VISA Write(VISA resource name=w587, write buffer=w593, error in (no error)=w586) -> (VISA resource name out=w584:refnum<visa-resource-name>, error out=w583:errorcluster)  [unwired: 1 out]
          }
          frame #11 {
            n261 = Wait (ms)(milliseconds to wait=u32 150) -> ()  [unwired: 1 out]
          }
          frame #12 {
            n262 = case shown="假" w598 {
              tunnel: w601 -> [w609 w610]
              tunnel: [w608 w617] -> w597
              tunnel: w600 -> [w607 w615]
              tunnel: [w606 w616] -> w599
              frame True {
                n263 = local write "Output"(TRUE ("布尔")) -> ()
                n264 = local read "channel输出口"() -> (w603:i32)
                n265 = Pick Line(multi-line string=":OUTP1 ON\n:OUTP2 ON" ("write buffer"), line index=w603) -> (output string=w602:string)  [unwired: 1 in]
                n266 = VISA Write(VISA resource name=w609, write buffer=w602, error in (no error)=w607) -> (VISA resource name out=w606:refnum<visa-resource-name>, error out=w608:errorcluster)  [unwired: 1 out]
              }
              frame False {
                n267 = local read "channel输出口"() -> (w612:i32)
                n268 = Pick Line(multi-line string=":OUTP1 OFF\n:OUTP2 OFF" ("write buffer"), line index=w612) -> (output string=w611:string)  [unwired: 1 in]
                n269 = VISA Write(VISA resource name=w610, write buffer=w611, error in (no error)=w615) -> (VISA resource name out=w616:refnum<visa-resource-name>, error out=w617:errorcluster)  [unwired: 1 out]
                n270 = local write "Output"(FALSE ("布尔")) -> ()
              }
            }
          }
        }
        n271 = VISA Close(VISA resource name=w520, error in (no error)=w519) -> (error out=→"output control error  4":errorcluster)
      }
    }
    n272 = event shown="[1] \"Enable\": 值改变" {
      selector: _ -> [_ _]
      dyn-events: _ -> [_ _]
      timeout: u32 0 ("Time") -> [_ _]
      tunnel: "Enable" -> [_ w493]
      event Timeout {
        n273 = event-data() -> ()  [unwired: 1 in, 2 out]
      }
      event "Enable": Value Change {
        n274 = event-data() -> ()  [unwired: 1 in, 6 out]
        n275 = local read "VISA 信号发生器"() -> (w489:refnum<visa-resource-name>)
        n276 = VISA Open(VISA resource name=w489) -> (VISA resource name=w492:refnum<visa-resource-name>, error out=w495:errorcluster)  [unwired: 4 in]
        n277 = stacked-sequence {
          tunnel: w493 -> [w500 _]
          tunnel: w495 -> [w499 _]
          tunnel: w492 -> [w498 _]
          tunnel: [w497 _] -> w491
          tunnel: [w496 _] -> w490
          frame #0 {
            n278 = case shown="真" w500 {
              tunnel: w498 -> [w508 w516]
              tunnel: [w507 w515] -> w496
              tunnel: w499 -> [w506 w513]
              tunnel: [w505 w514] -> w497
              frame True {
                n279 = local write "Output"(TRUE ("布尔")) -> ()
                n280 = local read "channel输出口"() -> (w502:i32)
                n281 = Pick Line(multi-line string=":OUTP1 ON\n:OUTP2 ON" ("write buffer"), line index=w502) -> (output string=w501:string)  [unwired: 1 in]
                n282 = VISA Write(VISA resource name=w508, write buffer=w501, error in (no error)=w506) -> (VISA resource name out=w505:refnum<visa-resource-name>, error out=w507:errorcluster)  [unwired: 1 out]
              }
              frame False {
                n283 = local read "channel输出口"() -> (w510:i32)
                n284 = Pick Line(multi-line string=":OUTP1 OFF\n:OUTP2 OFF" ("write buffer"), line index=w510) -> (output string=w509:string)  [unwired: 1 in]
                n285 = VISA Write(VISA resource name=w516, write buffer=w509, error in (no error)=w513) -> (VISA resource name out=w514:refnum<visa-resource-name>, error out=w515:errorcluster)  [unwired: 1 out]
                n286 = local write "Output"(FALSE ("布尔")) -> ()
              }
            }
          }
          frame #1 {
            n287 = Wait (ms)(milliseconds to wait=u32 150) -> ()  [unwired: 1 out]
          }
        }
        n288 = VISA Close(VISA resource name=w491, error in (no error)=w490) -> (error out=→"output control error  5":errorcluster)
      }
    }
    n289 = event shown="[1] \"Enable 2\": 值改变" {
      selector: _ -> [_ _]
      dyn-events: _ -> [_ _]
      timeout: u32 0 ("Time") -> [_ _]
      tunnel: "Enable 2" -> [_ w27]
      event Timeout {
        n290 = event-data() -> ()  [unwired: 1 in, 2 out]
      }
      event "Enable 2": Value Change {
        n291 = event-data() -> ()  [unwired: 1 in, 6 out]
        n292 = Not(x=w27) -> (.not. x?=w26:bool)
        n293 = local read "VISA 信号发生器"() -> (w28:refnum<visa-resource-name>)
        n294 = VISA Open(VISA resource name=w28) -> (VISA resource name=w31:refnum<visa-resource-name>, error out=w32:errorcluster)  [unwired: 4 in]
        n295 = stacked-sequence {
          tunnel: w26 -> [w37 _]
          tunnel: w32 -> [w36 _]
          tunnel: w31 -> [w35 _]
          tunnel: [w34 _] -> w30
          tunnel: [w33 _] -> w29
          frame #0 {
            n296 = case shown="真" w37 {
              tunnel: w35 -> [w46 w57]
              tunnel: [w45 w56] -> w33
              tunnel: w36 -> [w44 w54]
              tunnel: [w43 w55] -> w34
              frame True {
                n297 = local read "channel输出口"() -> (w39:i32)
                n298 = local write "Output 2"(FALSE ("布尔")) -> ()
                n299 = case shown="1" w39 {
                  tunnel: [1 0] -> w38
                  frame 0, Default {
                  }
                  frame 1 {
                  }
                }
                n300 = Pick Line(multi-line string=":OUTP1 ON\n:OUTP2 ON" ("write buffer"), line index=w38) -> (output string=w40:string)  [unwired: 1 in]
                n301 = VISA Write(VISA resource name=w46, write buffer=w40, error in (no error)=w44) -> (VISA resource name out=w43:refnum<visa-resource-name>, error out=w45:errorcluster)  [unwired: 1 out]
              }
              frame False {
                n302 = local read "channel输出口"() -> (w50:i32)
                n303 = case shown="1" w50 {
                  tunnel: [1 0] -> w49
                  frame 0, Default {
                  }
                  frame 1 {
                  }
                }
                n304 = Pick Line(multi-line string=":OUTP1 OFF\n:OUTP2 OFF" ("write buffer"), line index=w49) -> (output string=w51:string)  [unwired: 1 in]
                n305 = VISA Write(VISA resource name=w57, write buffer=w51, error in (no error)=w54) -> (VISA resource name out=w55:refnum<visa-resource-name>, error out=w56:errorcluster)  [unwired: 1 out]
                n306 = local write "Output 2"(TRUE ("布尔")) -> ()
              }
            }
          }
          frame #1 {
            n307 = Wait (ms)(milliseconds to wait=u32 150) -> ()  [unwired: 1 out]
          }
        }
        n308 = VISA Close(VISA resource name=w30, error in (no error)=w29) -> ()  [unwired: 1 out]
      }
    }
    n309 = case shown="真" "设置参数" {
      frame False {
      }
      frame True {
        w624 = " :SOUR1\n :SOUR2"  # Channel
        n310 = local read "VISA 信号发生器"() -> (w626:refnum<visa-resource-name>)
        n311 = local read "channel输出口"() -> (w625:i32)
        n312 = case shown="1" w625 {
          tunnel: [1 0] -> w618
          frame 0, Default {
          }
          frame 1 {
          }
        }
        n313 = VISA Open(VISA resource name=w626) -> (VISA resource name=w629:refnum<visa-resource-name>, error out=w630:errorcluster)  [unwired: 4 in]
        n314 = Pick Line(multi-line string=w624, line index=w618) -> (output string=w619:string)  [unwired: 1 in]
        n315 = Pick Line(multi-line string=w624, line index=w625) -> (output string=w627:string)  [unwired: 1 in]
        n316 = stacked-sequence {
          seq-local: [w726 _ _ _ _ _ _ _ _ _ _ _ _ _ _] -> [_ _ w741 _ _ _ _ _ _ _ _ _ _ _ _]
          seq-local: [w725 _ _ _ _ _ _ _ _ _ _ _ _ _ _] -> [_ _ w740 _ _ _ _ _ _ _ w779 _ _ _ _]
          seq-local: [_ _ w739 _ _ _ _ _ _ _ _ _ _ _ _] -> [_ _ _ _ w750 _ _ _ _ _ _ _ _ _ _]
          seq-local: [_ _ w738 _ _ _ _ _ _ _ _ _ _ _ _] -> [_ _ _ _ w749 _ _ _ _ _ _ _ _ _ _]
          seq-local: [_ _ _ _ w748 _ _ _ _ _ _ _ _ _ _] -> [_ _ _ _ _ _ w756 _ _ _ _ _ _ _ _]
          seq-local: [_ _ _ _ w745 _ _ _ _ _ _ _ _ _ _] -> [_ _ _ _ _ _ w755 _ _ _ _ _ _ _ _]
          seq-local: [_ _ _ _ _ _ w763 _ _ _ _ _ _ _ _] -> [_ _ _ _ _ _ _ _ w774 _ _ _ _ _ _]
          seq-local: [_ _ _ _ _ _ w762 _ _ _ _ _ _ _ _] -> [_ _ _ _ _ _ _ _ w773 _ _ _ _ _ _]
          seq-local: [_ _ _ _ _ _ _ _ w767 _ _ _ _ _ _] -> [_ _ _ _ _ _ _ _ _ _ w780 _ _ _ _]
          seq-local: [_ _ _ _ _ _ _ _ w766 _ _ _ _ _ _] -> [_ _ _ _ _ _ _ _ _ _ _ _ _ _ _]
          seq-local: [_ _ _ _ _ _ _ _ _ _ w776 _ _ _ _] -> [_ _ _ _ _ _ _ _ _ _ _ _ w790 _ _]
          seq-local: [_ _ _ _ _ _ _ _ _ _ w777 _ _ _ _] -> [_ _ _ _ _ _ _ _ _ _ _ _ w789 _ _]
          seq-local: [_ _ _ _ _ _ _ _ _ _ _ _ w788 _ _] -> [_ _ _ _ _ _ _ _ _ _ _ _ _ _ w801]
          seq-local: [_ _ _ _ _ _ _ _ _ _ _ _ w787 _ _] -> [_ _ _ _ _ _ _ _ _ _ _ _ _ _ w800]
          tunnel: w629 -> [w731 _ _ _ _ _ _ _ _ _ _ _ _ _ _]
          tunnel: w630 -> [w724 _ _ _ _ _ _ _ _ _ _ _ _ _ _]
          tunnel: w627 -> [w723 _ w737 _ w744 _ w760 _ w771 _ w781 _ w791 _ w804]
          tunnel: [_ _ _ _ _ _ _ _ _ _ _ _ _ _ w799] -> w623
          tunnel: [_ _ _ _ _ _ _ _ _ _ _ _ _ _ w798] -> w622
          frame #0 {
            w728 = " PULSe"  # Function Command
            n317 = local read "输出信号波形"() -> (w722:u16)
            n318 = Concatenate Strings(w723, ":FUNC" ("string (\"\")")) -> (w729:string)
            n319 = Pick Line(string ("")=w729, multi-line string=w728, line index=w722) -> (output string=w727:string)
            n320 = VISA Write(VISA resource name=w731, write buffer=w727, error in (no error)=w724) -> (VISA resource name out=w726:refnum<visa-resource-name>, error out=w725:errorcluster)  [unwired: 1 out]
          }
          frame #1 {
            n321 = Wait (ms)(milliseconds to wait=u32 150) -> ()  [unwired: 1 out]
          }
          frame #2 {
            n322 = Number To Fractional String(use system decimal point (T)=TRUE ("使用系统小数点(T)"), number="低电平/V") -> (F-format string=w735:string)  [unwired: 2 in]
            n323 = Concatenate Strings ("连接字符串")(w737, ":VOLTage:LOW ", w735) -> (w734:string)
            n324 = VISA Write(VISA resource name=w741, write buffer=w734, error in (no error)=w740) -> (VISA resource name out=w739:refnum<visa-resource-name>, error out=w738:errorcluster)  [unwired: 1 out]
          }
          frame #3 {
            n325 = Wait (ms)(milliseconds to wait=u32 150) -> ()  [unwired: 1 out]
          }
          frame #4 {
            # "1 频率"
            n326 = Concatenate Strings(w744, ":FREQ ") -> (w751:string)
            n327 = Format Into String ("格式化写入字符串")(initial string=w751, "频率/Hz") -> (resulting string=w752:string)  [unwired: 2 in, 1 out]
            n328 = VISA Write(VISA resource name=w750, write buffer=w752, error in (no error)=w749) -> (VISA resource name out=w748:refnum<visa-resource-name>, error out=w745:errorcluster)  [unwired: 1 out]
          }
          frame #5 {
            n329 = Wait (ms)(milliseconds to wait=u32 150) -> ()  [unwired: 1 out]
          }
          frame #6 {
            n330 = Number To Fractional String(use system decimal point (T)=TRUE ("使用系统小数点(T)"), number="高电平/V") -> (F-format string=w757:string)  [unwired: 2 in]
            n331 = Concatenate Strings(w760, ":VOLTage:HIGH ", w757) -> (w759:string)
            n332 = VISA Write(VISA resource name=w756, write buffer=w759, error in (no error)=w755) -> (VISA resource name out=w763:refnum<visa-resource-name>, error out=w762:errorcluster)  [unwired: 1 out]
          }
          frame #7 {
            n333 = Wait (ms)(milliseconds to wait=u32 150) -> ()  [unwired: 1 out]
          }
          frame #8 {
            n334 = local read "channel输出口"() -> (w769:i32)
            n335 = Pick Line(multi-line string=":OUTP1:IMPedance \n:OUTP2:IMPedance " ("write buffer"), line index=w769) -> (output string=w768:string)  [unwired: 1 in]
            n336 = Concatenate Strings ("连接字符串")(w771, w768, "INFINITY") -> (w772:string)
            n337 = VISA Write(VISA resource name=w774, write buffer=w772, error in (no error)=w773) -> (VISA resource name out=w767:refnum<visa-resource-name>, error out=w766:errorcluster)  [unwired: 1 out]
          }
          frame #9 {
            n338 = Wait (ms)(milliseconds to wait=u32 150) -> ()  [unwired: 1 out]
          }
          frame #10 {
            n339 = Number To Fractional String(use system decimal point (T)=TRUE ("使用系统小数点(T)"), number="占空比/%") -> (F-format string=w783:string)  [unwired: 2 in]
            n340 = Concatenate Strings(w781, ":PULSe:DCYCle ", w783) -> (w778:string)
            n341 = VISA Write(VISA resource name=w780, write buffer=w778, error in (no error)=w779) -> (VISA resource name out=w776:refnum<visa-resource-name>, error out=w777:errorcluster)  [unwired: 1 out]
          }
          frame #11 {
            n342 = Wait (ms)(milliseconds to wait=u32 150) -> ()  [unwired: 1 out]
          }
          frame #12 {
            n343 = Number To Fractional String(use system decimal point (T)=TRUE ("使用系统小数点(T)"), number="延时/s") -> (F-format string=w794:string)  [unwired: 2 in]
            n344 = Concatenate Strings(w791, ":PULSe:DELay ", w794) -> (w792:string)
            n345 = VISA Write(VISA resource name=w790, write buffer=w792, error in (no error)=w789) -> (VISA resource name out=w788:refnum<visa-resource-name>, error out=w787:errorcluster)  [unwired: 1 out]
          }
          frame #13 {
            n346 = Wait (ms)(milliseconds to wait=u32 150) -> ()  [unwired: 1 out]
          }
          frame #14 {
            w805 = ":LEADing\n:TRAiling "  # Channel
            w810 = ":PULSe:TRANsition"  # VOLTage:Offset
            n347 = local read "上升下降沿"() -> (w806:i32)
            n348 = Pick Line(multi-line string=w805, line index=w806) -> (output string=w802:string)  [unwired: 1 in]
            n349 = Number To Fractional String(use system decimal point (T)=TRUE ("使用系统小数点(T)"), number="上升下降沿/s") -> (F-format string=w803:string)  [unwired: 2 in]
            n350 = Concatenate Strings(w804, w810, w802, w803) -> (w807:string)
            n351 = VISA Write(VISA resource name=w801, write buffer=w807, error in (no error)=w800) -> (VISA resource name out=w799:refnum<visa-resource-name>, error out=w798:errorcluster)  [unwired: 1 out]
          }
        }
        n352 = stacked-sequence {
          seq-local: [w637 _ _ _ _ _ _ _ _ _ _ _ _ _ _] -> [_ _ w652 _ _ _ _ _ _ _ _ _ _ _ _]
          seq-local: [w636 _ _ _ _ _ _ _ _ _ _ _ _ _ _] -> [_ _ w651 _ _ _ _ _ _ _ w690 _ _ _ _]
          seq-local: [_ _ w650 _ _ _ _ _ _ _ _ _ _ _ _] -> [_ _ _ _ w661 _ _ _ _ _ _ _ _ _ _]
          seq-local: [_ _ w649 _ _ _ _ _ _ _ _ _ _ _ _] -> [_ _ _ _ w660 _ _ _ _ _ _ _ _ _ _]
          seq-local: [_ _ _ _ w659 _ _ _ _ _ _ _ _ _ _] -> [_ _ _ _ _ _ w667 _ _ _ _ _ _ _ _]
          seq-local: [_ _ _ _ w656 _ _ _ _ _ _ _ _ _ _] -> [_ _ _ _ _ _ w666 _ _ _ _ _ _ _ _]
          seq-local: [_ _ _ _ _ _ w674 _ _ _ _ _ _ _ _] -> [_ _ _ _ _ _ _ _ w685 _ _ _ _ _ _]
          seq-local: [_ _ _ _ _ _ w673 _ _ _ _ _ _ _ _] -> [_ _ _ _ _ _ _ _ w684 _ _ _ _ _ _]
          seq-local: [_ _ _ _ _ _ _ _ w679 _ _ _ _ _ _] -> [_ _ _ _ _ _ _ _ _ _ w691 _ _ _ _]
          seq-local: [_ _ _ _ _ _ _ _ w678 _ _ _ _ _ _] -> [_ _ _ _ _ _ _ _ _ _ _ _ _ _ _]
          seq-local: [_ _ _ _ _ _ _ _ _ _ w687 _ _ _ _] -> [_ _ _ _ _ _ _ _ _ _ _ _ w701 _ _]
          seq-local: [_ _ _ _ _ _ _ _ _ _ w688 _ _ _ _] -> [_ _ _ _ _ _ _ _ _ _ _ _ w700 _ _]
          seq-local: [_ _ _ _ _ _ _ _ _ _ _ _ w699 _ _] -> [_ _ _ _ _ _ _ _ _ _ _ _ _ _ w714]
          seq-local: [_ _ _ _ _ _ _ _ _ _ _ _ w698 _ _] -> [_ _ _ _ _ _ _ _ _ _ _ _ _ _ w713]
          tunnel: w623 -> [w642 _ _ _ _ _ _ _ _ _ _ _ _ _ _]
          tunnel: w622 -> [w635 _ _ _ _ _ _ _ _ _ _ _ _ _ _]
          tunnel: w619 -> [w634 _ w648 _ w655 _ w671 _ w682 _ w692 _ w702 _ w709]
          tunnel: [_ _ _ _ _ _ _ _ _ _ _ _ _ _ w712] -> w621
          tunnel: [_ _ _ _ _ _ _ _ _ _ _ _ _ _ w711] -> w620
          tunnel: w618 -> [_ _ _ _ _ _ _ _ w676 _ _ _ _ _ _]
          frame #0 {
            w639 = " PULSe"  # Function Command
            n353 = Concatenate Strings(w634, ":FUNC" ("string (\"\")")) -> (w640:string)
            n354 = Pick Line(string ("")=w640, multi-line string=w639, line index="输出信号波形 2") -> (output string=w638:string)
            n355 = VISA Write(VISA resource name=w642, write buffer=w638, error in (no error)=w635) -> (VISA resource name out=w637:refnum<visa-resource-name>, error out=w636:errorcluster)  [unwired: 1 out]
          }
          frame #1 {
            n356 = Wait (ms)(milliseconds to wait=u32 150) -> ()  [unwired: 1 out]
          }
          frame #2 {
            n357 = Number To Fractional String(use system decimal point (T)=TRUE ("使用系统小数点(T)"), number="低电平/V 2") -> (F-format string=w646:string)  [unwired: 2 in]
            n358 = Concatenate Strings ("连接字符串")(w648, ":VOLTage:LOW ", w646) -> (w645:string)
            n359 = VISA Write(VISA resource name=w652, write buffer=w645, error in (no error)=w651) -> (VISA resource name out=w650:refnum<visa-resource-name>, error out=w649:errorcluster)  [unwired: 1 out]
          }
          frame #3 {
            n360 = Wait (ms)(milliseconds to wait=u32 150) -> ()  [unwired: 1 out]
          }
          frame #4 {
            # "1 频率"
            n361 = Concatenate Strings(w655, ":FREQ ") -> (w662:string)
            n362 = Format Into String ("格式化写入字符串")(initial string=w662, "频率/Hz 2") -> (resulting string=w663:string)  [unwired: 2 in, 1 out]
            n363 = VISA Write(VISA resource name=w661, write buffer=w663, error in (no error)=w660) -> (VISA resource name out=w659:refnum<visa-resource-name>, error out=w656:errorcluster)  [unwired: 1 out]
          }
          frame #5 {
            n364 = Wait (ms)(milliseconds to wait=u32 150) -> ()  [unwired: 1 out]
          }
          frame #6 {
            n365 = Number To Fractional String(use system decimal point (T)=TRUE ("使用系统小数点(T)"), number="高电平/V 2") -> (F-format string=w668:string)  [unwired: 2 in]
            n366 = Concatenate Strings(w671, ":VOLTage:HIGH ", w668) -> (w670:string)
            n367 = VISA Write(VISA resource name=w667, write buffer=w670, error in (no error)=w666) -> (VISA resource name out=w674:refnum<visa-resource-name>, error out=w673:errorcluster)  [unwired: 1 out]
          }
          frame #7 {
            n368 = Wait (ms)(milliseconds to wait=u32 150) -> ()  [unwired: 1 out]
          }
          frame #8 {
            n369 = Pick Line(multi-line string=":OUTP1:IMPedance \n:OUTP2:IMPedance " ("write buffer"), line index=w676) -> (output string=w680:string)  [unwired: 1 in]
            n370 = Concatenate Strings ("连接字符串")(w682, w680, "INFINITY") -> (w683:string)
            n371 = VISA Write(VISA resource name=w685, write buffer=w683, error in (no error)=w684) -> (VISA resource name out=w679:refnum<visa-resource-name>, error out=w678:errorcluster)  [unwired: 1 out]
          }
          frame #9 {
            n372 = Wait (ms)(milliseconds to wait=u32 150) -> ()  [unwired: 1 out]
          }
          frame #10 {
            n373 = Number To Fractional String(use system decimal point (T)=TRUE ("使用系统小数点(T)"), number="占空比/% 2") -> (F-format string=w694:string)  [unwired: 2 in]
            n374 = Concatenate Strings(w692, ":PULSe:DCYCle ", w694) -> (w689:string)
            n375 = VISA Write(VISA resource name=w691, write buffer=w689, error in (no error)=w690) -> (VISA resource name out=w687:refnum<visa-resource-name>, error out=w688:errorcluster)  [unwired: 1 out]
          }
          frame #11 {
            n376 = Wait (ms)(milliseconds to wait=u32 150) -> ()  [unwired: 1 out]
          }
          frame #12 {
            n377 = Number To Fractional String(use system decimal point (T)=TRUE ("使用系统小数点(T)"), number="延时/s 2") -> (F-format string=w705:string)  [unwired: 2 in]
            n378 = Concatenate Strings(w702, ":PULSe:DELay ", w705) -> (w703:string)
            n379 = VISA Write(VISA resource name=w701, write buffer=w703, error in (no error)=w700) -> (VISA resource name out=w699:refnum<visa-resource-name>, error out=w698:errorcluster)  [unwired: 1 out]
          }
          frame #13 {
            n380 = Wait (ms)(milliseconds to wait=u32 150) -> ()  [unwired: 1 out]
          }
          frame #14 {
            w717 = ":LEADing\n:TRAiling "  # Channel
            w721 = ":PULSe:TRANsition"  # VOLTage:Offset
            n381 = Pick Line(multi-line string=w717, line index="上升下降沿 2") -> (output string=w715:string)  [unwired: 1 in]
            n382 = Number To Fractional String(use system decimal point (T)=TRUE ("使用系统小数点(T)"), number="上升下降沿/s 2") -> (F-format string=w716:string)  [unwired: 2 in]
            n383 = Concatenate Strings(w709, w721, w715, w716) -> (w718:string)
            n384 = VISA Write(VISA resource name=w714, write buffer=w718, error in (no error)=w713) -> (VISA resource name out=w712:refnum<visa-resource-name>, error out=w711:errorcluster)  [unwired: 1 out]
          }
        }
        n385 = VISA Close(VISA resource name=w621, error in (no error)=w620) -> (error out=→"configure error out":errorcluster)
      }
    }
    n386 = event shown="[1] \"照明光\": 值改变" {
      selector: _ -> [_ _]
      dyn-events: _ -> [_ _]
      timeout: 0 -> [_ _]
      tunnel: "照明光" -> [_ w61]
      event Timeout {
        n387 = event-data() -> ()  [unwired: 1 in, 3 out]
      }
      event "照明光": Value Change {
        n388 = event-data() -> ()  [unwired: 1 in, 6 out]
        n389 = local read "stop bits (10: 1 bit)"() -> (w74:u16)
        n390 = local read "parity (0:none)"() -> (w73:enum16{"None", "Odd", "Even", "Mark", "Space"})
        n391 = local read "照明光VISA"() -> (w70:refnum<visa-resource-name>)
        n392 = local read "baud rate"() -> (w71:u32)
        n393 = local read "data bits (8)"() -> (w72:u16)
        n394 = call-poly "VISA Configure Serial Port"("VISA resource name"=w70, "baud rate (9600)"=w71, "data bits (8)"=w72, "parity (0:none)"=w73, "stop bits (10: 1 bit)"=w74) -> ("VISA resource name out"=w67:refnum<visa-resource-name>, "error out"=w66:errorcluster)  [unwired: 9 in]
        n395 = call <vilib>:"Simple Error Handler.vi"("error in (no error)"=w66) -> ()  [unwired: 4 in, 5 out]
        n396 = VISA Open(access mode=0, error in (no error)=w66, VISA resource name=w67) -> (VISA resource name=w69:refnum<visa-resource-name>, error out=w68:errorcluster)  [unwired: 2 in]
        n397 = stacked-sequence {
          tunnel: w69 -> [w79]
          tunnel: w68 -> [w78]
          tunnel: [w77] -> w64
          tunnel: [w76] -> w65
          tunnel: w61 -> [w75]
          frame #0 {
            n398 = case shown="假" w75 {
              tunnel: w79 -> [w85 w95]
              tunnel: [w83 w94] -> w77
              tunnel: w78 -> [w84 w93]
              tunnel: [w82 w92] -> w76
              frame False {
                n399 = Concatenate Strings(" \u0001\u0001¢", "\r") -> (w86:string)
                n400 = VISA Write(VISA resource name=w85, write buffer=w86, error in (no error)=w84) -> (VISA resource name out=w83:refnum<visa-resource-name>, error out=w82:errorcluster)  [unwired: 1 out]
                n401 = Wait (ms)(milliseconds to wait=50) -> ()  [unwired: 1 out]
              }
              frame True {
                w88 = " \u0001\u0000¡"  # Channel
                n402 = Wait (ms)(milliseconds to wait=50) -> ()  [unwired: 1 out]
                n403 = Concatenate Strings(w88, "\r") -> (w89:string)
                n404 = VISA Write(VISA resource name=w95, write buffer=w89, error in (no error)=w93) -> (VISA resource name out=w94:refnum<visa-resource-name>, error out=w92:errorcluster)  [unwired: 1 out]
              }
            }
          }
        }
        n405 = VISA Close(VISA resource name=w64, error in (no error)=w65) -> (error out=w63:errorcluster)
        n406 = call <vilib>:"Simple Error Handler.vi"("error in (no error)"=w63) -> ()  [unwired: 4 in, 5 out]
      }
    }
  }
  n407 = flat-sequence {
    frame #0 {
      "Backlight" <- i32[][] [] ("Backlight")
    }
    frame #1 {
      w812 = FALSE
      # "删除背景光控件\n初始值设定"
      n408 = local write "cut backlight"(w812) -> ()
      "backlight" <- w812
    }
  }
  n409 = stacked-sequence {
    seq-local: [_ _ _ w833 _ _ _ _] -> [_ _ _ _ w851 w871 w874 w1076]
    seq-local: [_ _ _ w832 _ _ _ _] -> [_ _ _ _ w852 w872 w873 w1077]
    frame #0 {
      # "initialize all variables"
      n410 = property on="initialize" class="Bool"("Désactivé"=u8 0) -> ()  [unwired: 2 in, 2 out]
      n411 = property on="Acquire" class="Bool"("Visible"=FALSE) -> ()  [unwired: 2 in, 2 out]
      n412 = property on="Setup" class="Bool"("Visible"=FALSE) -> ()  [unwired: 2 in, 2 out]
      n413 = local write "indicator"("" ("indicator")) -> ()
      n414 = local write "initialized ?"(FALSE ("initialized ?")) -> ()
      n415 = local write "Continuous"(FALSE ("Continuous")) -> ()
      n416 = local write "Close"(FALSE ("Close")) -> ()
      n417 = property on="Device Name" class="Ring (严格)"("Désactivé"=u8 0) -> ()  [unwired: 2 in, 2 out]
      n418 = property on="Continuous" class="Bool (严格)"("Visible"=FALSE) -> ()  [unwired: 2 in, 2 out]
      n419 = local write "Commande tab"(T1."Settings" ("Commande tab")) -> ()
    }
    frame #1 {
      # "Read Uniq ID"
      n420 = stacked-sequence {
        frame #0 {
          n421 = call "read detector uniq-id.vi"() -> ("nbr of components"=w825:i32, "UniqueID"=w824:string[], "Name"=w823:string[])  [unwired: 4 out]
          n422 = for {
            N: w825 -> [_]
            tunnel: w824 -> [w827]
            tunnel: w823 -> [w826]
            n423 = property on="Device Name" class="Ring (严格)"("Chaînes []"=w826) -> ()  [unwired: 2 in, 2 out]
            n424 = property on="Uniques ID" class="Ring (严格)"("Chaînes []"=w827) -> ()  [unwired: 2 in, 2 out]
          }
        }
      }
    }
    frame #2 {
      n425 = while {
        stop <- "initialize" stop-if-true
        n426 = local read "Device Name"() -> (w830:u16)
        n427 = local write "Uniques ID"(w830) -> ()
        n428 = local read "Close"() -> (w828:bool)
        n429 = Stop(stop? (T)=w828) -> ()
        n430 = Wait Until Next ms Multiple(millisecond multiple=u32 100 ("n millisecondes")) -> ()  [unwired: 1 out]
      }
    }
    frame #3 {
      n431 = stacked-sequence {
        tunnel: [_ w840 _ _] -> w833
        tunnel: [_ w839 _ _] -> w832
        frame #0 {
          n432 = local write "indicator"("Initializing ..." ("indicator")) -> ()
        }
        frame #1 {
          n433 = local read "Uniques ID"() -> (w837:u16)
          n434 = property on="Uniques ID" class="Ring (严格)"() -> ("Chaînes []"=w838:string[])  [unwired: 2 in, 2 out]
          n435 = Index Array(array=w838, index=w837) -> (element=w836:string)
          n436 = call "Initialize CCD.vi"("Unique id:"=w836) -> ("activeYPixels"=→"Y Pixels:":i32, "JYCCDLib.IJYCCDReqd"=w839:refnum<k7>, "activeXPixels"=→"X Pixels:":i32, "sortie d'erreur"=w840:errorcluster, "FirmwareVersion"=→"Firmware\nVersion":string)  [unwired: 3 out]
        }
        frame #2 {
          n437 = property on="initialize" class="Bool"("Désactivé"=u8 2) -> ()  [unwired: 2 in, 2 out]
          n438 = property on="Device Name" class="Ring (严格)"("Désactivé"=u8 2) -> ()  [unwired: 2 in, 2 out]
          n439 = local write "Continuous"(FALSE ("Continuous")) -> ()
          n440 = property on="Setup" class="Bool"("Visible"=TRUE) -> ()  [unwired: 2 in, 2 out]
        }
        frame #3 {
          n441 = local write "initialized ?"(TRUE ("initialized ?")) -> ()
          n442 = local write "indicator"("Initialized !" ("indicator")) -> ()
        }
      }
    }
    frame #4 {
      # "Actually not working"
      # "Read ADC and GAIN"
      n443 = case shown="真" "Constante de condition\n(Voir l'aide contextuelle)" {
        tunnel: w852 -> [_ w862]
        tunnel: w851 -> [_ w861]
        frame False {
        }
        frame True {
          # "Read Input supported trigger"
          n444 = call "Trigger - Get Supported Input.vi"("JYCCDLib.IJYCCDReqd"=w862, "Error Input"=w861) -> ("trigAddress"=w856:i32, "eventPtr"=w857:i32, "trigEventString"=w860:string, "trigSigType"=w859:i32, "trigSigTypeString"=w858:string)  [unwired: 4 out]
          n445 = local write "trigSigTypeString"(w858) -> ()
          n446 = local write "trigAddress"(w856) -> ()
          n447 = local write "Trigger Type :"(w857) -> ()
          n448 = local write "trigEventString"(w860) -> ()
          n449 = local write "Signal type :"(w859) -> ()
        }
      }
      n450 = call "Init ADC & Gain.vi"("JYCCDLib.IJYCCDReqd"=w852, "input error"=w851) -> ("ADC Number"=w850:i32[], "ADC description"=w855:string[], "Gain Number"=w853:i32[], "Gain description"=w854:string[])
      n451 = local write "Gain Number"(w853) -> ()
      n452 = local write "ADC Number"(w850) -> ()
      n453 = stacked-sequence {
        tunnel: w855 -> [w863 _]
        tunnel: w854 -> [_ w864]
        frame #0 {
          n454 = property on="ADC" class="Ring (严格)"("Chaînes []"=w863) -> ()  [unwired: 2 in, 2 out]
        }
        frame #1 {
          n455 = property on="GAIN" class="Ring (严格)"("Chaînes []"=w864) -> ()  [unwired: 2 in, 2 out]
        }
      }
    }
    frame #5 {
      # "IS multi Accumulation Supported ?"
      n456 = call "MultiAccu - Is Supported.vi"("Error In"=w871, "JYCCDLib.IJYCCDReqd"=w872) -> ("IsOperatingModeSupported"=w865:bool)  [unwired: 3 out]
      n457 = Select(t=0, s=w865, f=2) -> (s? t:f=w868:i32)
      n458 = Select(t=FALSE, s=w865, f=w865) -> (s? t:f=w867:bool)
      n459 = local write "Multi Accumulation mode:"(w867) -> ()
      n460 = property on="Multi Accumulation mode:" class="Bool (严格)"("Désactivé"=w868) -> ()  [unwired: 2 in, 2 out]
      n461 = property on="Multi Accumulation mode:" class="Bool (严格)"("Désactivé"=w868) -> ()  [unwired: 2 in, 2 out]
    }
    frame #6 {
      n462 = while {
        tunnel: w873 -> [w881]
        tunnel: w874 -> [w880]
        stop <- "Close" stop-if-true
        n463 = local read "Continuous"() -> (w882:bool)
        n464 = case shown="假" "Reformat" {
          frame False {
          }
          frame True {
            n465 = local read "Y Pixels:"() -> (w1054:i32)
            n466 = local read "X Pixels:"() -> (w1056:i32)
            n467 = call "Spectral Reformat CCD area.vi"("Y Pixels:"=w1054, "X Pixels:"=w1056, "numAreas"="Number of Areas :") -> ("areas :"=→"areas :":i32[][])  [unwired: 3 out]
          }
        }
        n468 = local read "Accumulations:"() -> (w877:u16)
        n469 = Or(x="Acquire", y=w882) -> (x .or. y?=w879:bool)
        n470 = case shown="真" w879 {
          tunnel: w881 -> [_ w894]
          tunnel: w880 -> [_ w893]
          tunnel: "Enable InputTriggers :" -> [_ w892]
          tunnel: "Multi Accumulation mode:" -> [_ w891]
          tunnel: w877 -> [_ w890]
          tunnel: "MultiAcqShutterMode" -> [_ w889]
          frame False {
          }
          frame True {
            n471 = stacked-sequence {
              seq-local: [_ _ w907 _ _] -> [_ _ _ w980 _]
              seq-local: [_ _ _ w953 _] -> [_ _ _ _ w1020]
              tunnel: w894 -> [_ w896 w911 w979 _]
              tunnel: w893 -> [_ w897 w910 w978 _]
              tunnel: w892 -> [_ w898 _ _ _]
              tunnel: w891 -> [_ _ w909 _ _]
              tunnel: w890 -> [_ _ w908 _ _]
              tunnel: w889 -> [_ _ w906 _ _]
              frame #0 {
                n472 = local write "CCD Busy"(TRUE ("CCD Busy")) -> ()
              }
              frame #1 {
                n473 = case shown="真" w898 {
                  tunnel: w897 -> [w899 w905]
                  tunnel: w896 -> [w900 w904]
                  frame False {
                    n474 = call "Trigger - Disable.vi"("Error In"=w899, "JYCCDLib.IJYCCDReqd"=w900) -> ()  [unwired: 6 out]
                  }
                  frame True {
                    n475 = local read "Trigger Type :"() -> (w901:u16)
                    n476 = local read "Signal type :"() -> (w902:enum16{"TTL Rising Edge", "TTL Falling Edge"})
                    n477 = local read "trigAddress"() -> (w903:i32)
                    n478 = call "Trigger - Enable.vi"("Error In"=w905, "sigType"=w902, "event"=w901, "trigAddress"=w903, "JYCCDLib.IJYCCDReqd"=w904) -> ()  [unwired: 3 out]
                  }
                }
              }
              frame #2 {
                n479 = case shown="真" w909 {
                  selector: w909 -> [_ w940]
                  tunnel: w911 -> [w937 w943]
                  tunnel: w910 -> [w936 w942]
                  tunnel: w908 -> [_ w941]
                  tunnel: [u16 1 ("Accumulations:") w941] -> w907
                  tunnel: w906 -> [_ w939]
                  frame False {
                    n480 = call "MultiAccu - Disable.vi"("Error In"=w936, "JYCCDLib.IJYCCDReqd"=w937) -> ()  [unwired: 4 out]
                  }
                  frame True {
                    n481 = call "MultiAccu - Configure.vi"("JYCCDLib.IJYCCDReqd"=w943, "Cleans Before"="Number of Cleans", "Accumulations:"=w941, "MultiAcqHardwareMode"=w940, "MultiAcqShutterMode"=w939, "Error In"=w942) -> ()  [unwired: 1 in, 9 out]
                  }
                }
                n482 = flat-sequence {
                  frame #0 {
                    n483 = Current VI's Path() -> (path=w917:path)
                    n484 = Get Date/Time In Seconds() -> (seconds since 1Jan1904=w919:timestamp)
                    n485 = Strip Path(path=w917) -> (stripped path=w918:path)  [unwired: 1 out]
                    n486 = Path To String(path=w918) -> (string=w920:string)
                    n487 = Format Date/Time String(time format string (%c)="%m.%d" ("时间格式字符串(%c)"), seconds (now)=w919) -> (date/time string=w926:string)  [unwired: 1 in]
                    n488 = Concatenate Strings(w920, "\\Save\\" ("字符串"), w926) -> (w921:string)
                    n489 = String To Path(string=w921) -> (path=w922:path)
                    n490 = call <vilib>:"Check if File or Folder Exists.vi"("path"=w922) -> ("file or folder exists?"=w923:bool, "dup path"=w925:path)  [unwired: 8 in, 1 out]
                    n491 = case shown="真" w923 {
                      tunnel: [w933 w934] -> w924
                      tunnel: w925 -> [w932 w934]
                      tunnel: w926 -> [w931 _]
                      frame False {
                        n492 = Create Folder(prompt (Create Folder)=w931, path (use dialog)=w932) -> (created path=w933:path)  [unwired: 1 in, 2 out]
                      }
                      frame True {
                      }
                    }
                    n493 = Format Date/Time String(time format string (%c)="%y%m%d%H%M%S " ("时间格式字符串(%c)"), seconds (now)=w919) -> (date/time string=w929:string)  [unwired: 1 in]
                    n494 = Path To String(path=w924) -> (string=w927:string)
                    n495 = Concatenate Strings(w927, "\\" ("字符串")) -> (w928:string)
                    n496 = Concatenate Strings(w928, w929) -> (w916:string)
                    n497 = String To Path(string=w916) -> (path=→"最终存储路径 2":path)
                  }
                }
              }
              frame #3 {
                n498 = local read "cut backlight"() -> (w967:bool)
                n499 = local read "backlight"() -> (w966:bool)
                n500 = call "MultiAccu - Acquire spectral.vi"("error in"=w978, "Accumulations:"=w980, "ShutterOpen"="ShutterOpen", "JYCCDLib.IJYCCDReqd"=w979) -> ("Acq Time(ms)"=→"Acq Time(ms)":u32, "Array Out"=w977:i32[][][])  [unwired: 1 out]
                n501 = And(x=w967, y=w966) -> (x .and. y?=w968:bool)
                n502 = call "Array reset dimension.vi"("Area Number"="Area Number to Display", "Array In"=w977) -> ("Array Out"=w969:i32[][])
                n503 = case shown="真" w968 {
                  tunnel: [w1016 w1017] -> w970
                  tunnel: w969 -> [w1016 w1018]
                  frame False {
                  }
                  frame True {
                    n504 = local read "Backlight"() -> (w1019:i32[][])
                    n505 = Subtract(x=w1018, y=w1019) -> (x-y=w1017:i32[][])
                  }
                }
                n506 = local read "波长范围"() -> (w945:dbl[])
                n507 = local write "Data"(w969) -> ()
                n508 = Index Array(array=w970, index (row)=0 ("禁用的索引 (列)")) -> (element=w971:i32[])  [unwired: 1 in]
                n509 = Reverse 1D Array(array=w971) -> (reversed array=w954:i32[])
                n510 = call "转换至动态数据2"("Array"=w945) -> ("Dynamic Data Type"=w973:dynamicdata)  [unwired: 3 in]
                n511 = call "转换至动态数据"("Array"=w954) -> ("Dynamic Data Type"=w974:dynamicdata)  [unwired: 3 in]
                n512 = call <vilib>:"Median Filter.vi"("left rank"=6, "X"=w954) -> ("Filtered X"=w959:dbl[])  [unwired: 8 in, 1 out]
                n513 = call "Build XY Graph2"("Y Input"=w974, "X Input"=w973) -> ("XY Graph"=w972:cluster{"Y":dbl[], "Y":dbl[]}[])  [unwired: 8 in, 1 out]
                n514 = Subtract(x="拟合终点", y="拟合起点") -> (x-y=w948:i32)
                n515 = local write "Spectrum"(w972) -> ()
                n516 = local read "滤波阈值"() -> (w963:dbl)
                n517 = Array Subset(array=w945, index="拟合起点", length=w948) -> (w951:dbl[])
                n518 = local read "拟合参数"() -> (w944:dbl[])
                n519 = In Range and Coerce(upper limit=w963, x=w959, lower limit=-100.0) -> (In Range?=w962:bool[])  [unwired: 1 out]
                n520 = Not(x=w962) -> (.not. x?=w956:bool[])
                n521 = local read "滤波阈值"() -> (w958:dbl)
                n522 = local write "范围内？"(w962) -> ()
                n523 = local read "X Pixels:"() -> (w960:i32)
                n524 = Or Array Elements(Boolean array=w956) -> (logical OR=w961:bool)
                n525 = case shown="真" w961 {
                  tunnel: w960 -> [_ w1003]
                  tunnel: w959 -> [w999 w1002]
                  tunnel: [w999 w1001] -> w947
                  tunnel: w958 -> [_ w1000]
                  frame False {
                  }
                  frame True {
                    n526 = for {
                      N: w1003 -> [_]
                      tunnel: w1002 -> [w1007] mode=indexing
                      tunnel: [w1006] -> w1001 mode=indexing
                      shift-right: [w1006] -> _
                      shift-left: _ -> [w1005]
                      tunnel: w1000 -> [w1004]
                      n527 = Greater?(x=w1007, y=w1004) -> (0:w1009:bool)
                      n528 = Less?(x=w1007, y=-100.0) -> (x < y?=w1010:bool)
                      n529 = Or(x=w1009, y=w1010) -> (x .or. y?=w1008:bool)
                      n530 = case shown="真" w1008 {
                        tunnel: w1007 -> [w1012 _]
                        tunnel: [w1012 w1014] -> w1006
                        tunnel: w1005 -> [_ w1015]
                        frame False {
                        }
                        frame True {
                          n531 = call <vilib>:"Median Filter PtByPt.vi"("rank"=5, "x"=w1015) -> ("Filtered x"=w1014:dbl)  [unwired: 2 in, 1 out]
                        }
                      }
                    }
                  }
                }
                n532 = Array Subset(array=w947, index="拟合起点", length=w948) -> (w950:dbl[])
                n533 = Bundle("波长范围"=w945, "Filtered X"=w947) -> (w946:cluster{"波长范围 ":dbl[], "Filtered X":dbl[]})  [unwired: 1 in]
                n534 = case shown="真" "是否拟合" {
                  tunnel: w950 -> [w983 w989]
                  tunnel: w951 -> [_ w988]
                  tunnel: [w983 w987] -> w965
                  tunnel: w946 -> [_ w985]
                  frame False {
                  }
                  frame True {
                    n535 = call "转换至动态数据7"("Array"=w989) -> ("Dynamic Data Type"=w994:dynamicdata)  [unwired: 3 in]
                    n536 = call "转换至动态数据8"("Array"=w988) -> ("Dynamic Data Type"=w995:dynamicdata)  [unwired: 3 in]
                    n537 = call "曲线拟合2"("Locations"=w995, "Signals"=w994) -> ("best fit"=w992:dynamicdata, "non-linear coefficients"=w993:dynamicdata)  [unwired: 5 in, 3 out]
                    n538 = call "从动态数据转换3"("Dynamic Data Type"=w993) -> ("Array"=w996:dbl[])  [unwired: 3 in]
                    n539 = call "从动态数据转换4"("Dynamic Data Type"=w992) -> ("Array"=w987:dbl[])  [unwired: 3 in]
                    n540 = Index Array(array=w996, index #1=0 ("索引"), index #2=1 ("索引")) -> (element #1=w998:dbl, element #2=w997:dbl)
                    n541 = local write "拟合参数"(w996) -> ()
                    n542 = local write "xc"(w998) -> ()
                    n543 = Bundle(w988, "Array"=w987) -> (w986:cluster{dbl[], "Array":dbl[]})  [unwired: 1 in]
                    n544 = local write "w"(w997) -> ()
                    n545 = Build Array(w985, w986) -> (→"best fit":cluster{"波长范围 ":dbl[], "Array":dbl[]}[])
                  }
                }
                n546 = Build Array(w951, w954, w965, w944) -> (w953:dbl[][])
              }
              frame #4 {
                n547 = case shown="真" "是否保存" {
                  tunnel: w1020 -> [_ w1024]
                  frame False {
                  }
                  frame True {
                    n548 = Get Date/Time In Seconds() -> (seconds since 1Jan1904=w1038:timestamp)
                    n549 = Get Date/Time String(date format (0)=enum16{"short", "long", "abbreviated"}."abbreviated" ("日期格式(0)"), seconds (now)=w1038, want seconds? (F)=TRUE ("需要秒？(F)")) -> (date string=w1036:string, time string=w1037:string)
                    n550 = Search and Replace String(replace all?=TRUE ("替换全部？(F)"), input string=w1037, search string=":" ("搜索字符串"), replace string="-" ("替换字符串(\"\")")) -> (result string=w1035:string)  [unwired: 4 in, 3 out]
                    n551 = local read "最终存储路径 2"() -> (w1039:path)
                    n552 = Path To String(path=w1039) -> (string=w1042:string)
                    n553 = Concatenate Strings(w1042, w1036, w1035, "光谱" ("字符串"), ".xls" ("字符串")) -> (w1041:string)
                    n554 = String To Path(string=w1041) -> (path=w1040:path)
                    n555 = call-poly <vilib>:"Write Delimited Spreadsheet.vi"("file path (dialog if empty)"=w1040, "format (%.3f)"="%.16f", "2D data"=w1024, "append to file? (new file:F)"=TRUE ("append to file? (F)"), "transpose? (no:F)"=TRUE ("transpose? (F)")) -> ()  [unwired: 9 in, 2 out]
                  }
                }
                n556 = case shown="真" "Save Backlight" {
                  frame False {
                  }
                  frame True {
                    w1043 = TRUE ("删除背景光")
                    n557 = local read "Data"() -> (w1045:i32[][])
                    n558 = local write "Backlight"(w1045) -> ()
                    n559 = local write "cut backlight"(w1043) -> ()
                    n560 = local write "backlight"(w1043) -> ()
                    n561 = local write "Save Backlight"(FALSE ("Save Backlight")) -> ()
                  }
                }
                n562 = local write "CCD Busy"(FALSE ("CCD Busy")) -> ()
              }
            }
          }
        }
        n563 = case shown="假" "Setup" {
          tunnel: w880 -> [_ w1059]
          tunnel: w881 -> [_ w1058]
          frame False {
          }
          frame True {
            n564 = stacked-sequence {
              tunnel: w1059 -> [_ w1073 _]
              tunnel: w1058 -> [_ w1061 _]
              frame #0 {
                n565 = local write "indicator"("Setting up the detector" ("indicator")) -> ()
              }
              frame #1 {
                w1071 = 1 items=["JYMCD_ACQ_FORMAT_IMAGE", "JYMCD_ACQ_FORMAT_SCAN"] ("Acquisition type")
                n566 = local read "Gain Number"() -> (w1066:i32[])
                n567 = local read "GAIN"() -> (w1062:u16)
                n568 = local read "ADC Number"() -> (w1067:i32[])
                n569 = local read "ADC"() -> (w1063:u16)
                n570 = Index Array(array=w1066, index=w1062) -> (element=w1064:i32)
                n571 = Index Array(array=w1067, index=w1063) -> (element=w1065:i32)
                n572 = local read "Number of Areas :"() -> (w1069:u16)
                n573 = local read "areas :"() -> (w1070:i32[][])
                n574 = call "Setup CCD.vi"("numAreas"=w1069, "areas :"=w1070, "JYCCDLib.IJYCCDReqd"=w1061, "entrée d'erreur (pas d'erreur)"=w1073, "Acquisition type"=w1071, "Gain"=w1064, "Select ADC"=w1065, "Integration time(ms)"="Integration time (ms) :") -> ("DataSize"=→"DataSize":i32)  [unwired: 1 out]
                "JYCCDLib.IJYCCDReqd" <- w1061
              }
              frame #2 {
                w1074 = TRUE ("Visible")
                n575 = property on="Continuous" class="Bool (严格)"("Visible"=w1074) -> ()  [unwired: 2 in, 2 out]
                n576 = property on="Acquire" class="Bool"("Visible"=w1074) -> ()  [unwired: 2 in, 2 out]
                n577 = local write "indicator"("Ready !" ("indicator")) -> ()
              }
            }
          }
        }
        n578 = case shown="假" "Temperature" {
          tunnel: w881 -> [_ w1048]
          tunnel: w880 -> [_ w1047]
          frame False {
            n579 = property on="temp graph" class="WFChart (严格)"("Visible"=FALSE) -> ()  [unwired: 2 in, 2 out]
          }
          frame True {
            n580 = stacked-sequence {
              tunnel: w1048 -> [_ w1053]
              tunnel: w1047 -> [_ w1052]
              frame #0 {
                n581 = property on="temp graph" class="WFChart (严格)"("Visible"=TRUE) -> ()  [unwired: 2 in, 2 out]
              }
              frame #1 {
                w1051 = u16 0 items=["° Celsius", "Kelvin", "° Farenheit"] ("units")
                n582 = call "read temperature.vi"("entrée d'erreur (pas d'erreur)"=w1052, "units"=w1051, "JYCCDLib.IJYCCDReqd"=w1053) -> ("Current Temperature"=w1050:dbl)
                n583 = local write "temp graph"(w1050) -> ()
              }
            }
          }
        }
        n584 = Wait Until Next ms Multiple(millisecond multiple=u32 50 ("n millisecondes")) -> ()  [unwired: 1 out]
      }
    }
    frame #7 {
      n585 = Close Reference(reference=w1077, error in (no error)=w1076) -> ()  [unwired: 1 out]
    }
  }
  n586 = stacked-sequence {
    seq-local: [_ _ w1087 _ _] -> [_ _ _ w1097 w1102]
    seq-local: [_ _ w1086 _ _] -> [_ _ _ w1096 _]
    seq-local: [_ _ _ w1095 _] -> [_ _ _ _ _]
    frame #0 {
      n587 = call "Get Monos From Config Browser.vi"() -> ("UniqueIDs"=w1082:string[], "Mono ID"=w1083:string[])  [unwired: 3 in, 1 out]
      n588 = Build Cluster Array(w1083, w1082) -> (w1080:cluster{"String":string, "String":string}[])
      n589 = property on="Mono ID" class="CmbBox"("Strings And Values []"=w1080) -> ()  [unwired: 2 in, 2 out]
      n590 = Index Array(array=w1080, index=0) -> (element=w1081:cluster{"String":string, "String":string})
      n591 = Unbundle(w1081) -> ("String"=w1078:string)  [unwired: 1 out]
      "Current UniqueID" <- w1078
      n592 = local write "Mono ID"(w1078) -> ()
    }
    frame #1 {
      n593 = while {
        stop <- "Connect" stop-if-true
        n594 = local read "Mono ID"() -> (w1084:string)
        n595 = local write "Current UniqueID"(w1084) -> ()
      }
    }
    frame #2 {
      n596 = local read "Mono ID"() -> (w1089:string)
      n597 = call "JYInitMono.vi"("Unique ID"=w1089, "Force Init"="Force\nInitialization") -> ("Refnum out"=w1087:refnum<k7>, "Initialized"=→"Initialized JY":bool, "error out"=w1086:errorcluster)  [unwired: 9 in, 2 out]
    }
    frame #3 {
      n598 = call "Show Current Grating.vi"("Refnum in"=w1097, "error in (no error)"=w1096) -> ("Gratings"=w1098:dbl[], "Grating Index"=w1092:i32, "Current Grating"=w1094:dbl, "Current Description"=w1091:string, "error out"=w1095:errorcluster)  [unwired: 5 in, 4 out]
      "Gratings" <- w1098
      n599 = local write "Current Grating"(w1094) -> ()
      n600 = local write "Current Description"(w1091) -> ()
      n601 = Number To Decimal String(number=w1098) -> (decimal integer string=w1100:string[])  [unwired: 1 in]
      n602 = Number To Decimal String(number=w1092) -> (decimal integer string=w1093:string)  [unwired: 1 in]
      n603 = property on="Target Grating" class="CmbBox"("Value"=w1093) -> ()  [unwired: 2 in, 2 out]
      n604 = Build Cluster Array(w1100, string[] ["1", "2", "3"]) -> (w1101:cluster{"Numeric":string, string}[])
      n605 = property on="Target Grating" class="CmbBox"("Strings And Values []"=w1101) -> ()  [unwired: 2 in, 2 out]
    }
    frame #4 {
      n606 = while {
        tunnel: w1102 -> [w1104]
        stop <- w1103 stop-if-true
        n607 = stacked-sequence {
          seq-local: [w1108 _ _ _ _] -> [_ w1115 w1126 _ w1134]
          seq-local: [w1107 _ _ _ _] -> [_ w1114 w1125 _ _]
          seq-local: [_ w1113 _ _ _] -> [_ _ _ _ _]
          seq-local: [_ w1112 _ _ _] -> [_ _ _ _ _]
          seq-local: [_ _ w1118 _ _] -> [_ _ _ _ _]
          seq-local: [_ _ w1117 _ _] -> [_ _ _ w1128 _]
          tunnel: w1104 -> [w1106 _ _ w1129 _]
          frame #0 {
            n608 = call "Show Current Grating.vi"("Refnum in"=w1106) -> ("Grating Index"=→"Grating Index":i32, "Current Grating"=→"Current Grating":dbl, "Current Description"=→"Current Description":string, "error out"=w1107:errorcluster, "JYMONOLib.IJYMonoReqd"=w1108:refnum<k7>)  [unwired: 6 in, 4 out]
          }
          frame #1 {
            n609 = call "JYGetCurrentWL.vi"("error in (no error)"=w1114, "JYMONOLib.IJYMonoReqd"=w1115) -> ("error out"=w1112:errorcluster, "Units"=→"Units":string, "Current WL"=→"Current WL":dbl, "JYMONOLib.IJYMonoReqd 2"=w1113:refnum<k7>)  [unwired: 6 in]
          }
          frame #2 {
            w1123 = u16 1 items=["Entrance", "Exit"] ("Mirror Number")
            w1124 = u16 0 items=["Entrance", "Exit"] ("Mirror Number")
            n610 = call "JYGetMirrorPos.vi"("error in (no error)"=w1125, "Mirror"=w1124, "Refnum In"=w1126) -> ("error out"=w1121:errorcluster, "Current Mirror Position"=→"Entrance Mirror\nPosition":i32, "Refnum Out"=w1122:refnum<k7>)  [unwired: 1 in]
            n611 = call "JYGetMirrorPos.vi"("error in (no error)"=w1121, "Mirror"=w1123, "Refnum In"=w1122) -> ("error out"=w1117:errorcluster, "Current Mirror Position"=→"Exit Mirror\nPosition":i32, "Refnum Out"=w1118:refnum<k7>)  [unwired: 1 in]
          }
          frame #3 {
            w1131 = u16 0 items=["Front Entrance", "Side Entrance", "Front Exit", "Side Exit", "First Intermediate", "Second Intermediate"] ("Slit")
            n612 = call "JYGetSlits.vi"("MonoRefNum IN"=w1129, "Slit"=w1131, "error in (no error)"=w1128) -> ("Units"=→"Units 2":string, "Slit Width"=→"Front Entrance":dbl, "error out"=→"error out":errorcluster)  [unwired: 13 in, 1 out]
          }
          frame #4 {
            n613 = case shown="假" "Move To\nTarget Positions" {
              tunnel: w1134 -> [_ w1135]
              frame False {
              }
              frame True {
                n614 = stacked-sequence {
                  seq-local: [w1137 _ _ _] -> [_ w1143 _ _]
                  seq-local: [_ w1141 _ _] -> [_ _ w1158 _]
                  seq-local: [_ _ w1145 _] -> [_ _ _ w1164]
                  seq-local: [_ _ _ w1161] -> [_ _ _ _]
                  tunnel: w1135 -> [w1139 w1142 w1156 w1165]
                  frame #0 {
                    n615 = property on="Target Grating" class="CmbBox"() -> ("Value"=w1136:string)  [unwired: 2 in, 2 out]
                    n616 = local read "error out"() -> (w1138:errorcluster)
                    n617 = Decimal String To Number(string=w1136) -> (number=w1140:i32)  [unwired: 2 in, 1 out]
                    n618 = call "JYTurret.vi"("error in (no error)"=w1138, "Grating Index"=w1140, "JYMONOLib.IJYMonoReqd"=w1139) -> ("error out"=w1137:errorcluster)  [unwired: 2 out]
                  }
                  frame #1 {
                    # "Move Grating to Target Position"
                    n619 = call "JYMoveToWavelength.vi"("error in (no error)"=w1143, "Target WL"="Target WL", "RefNum In"=w1142) -> ("error out"=w1141:errorcluster)  [unwired: 1 in, 2 out]
                  }
                  frame #2 {
                    w1151 = u16 1 items=["Entrance", "Exit"] ("Mirror Number")
                    w1150 = u16 0 items=["Entrance", "Exit"] ("Mirror Number")
                    w1157 = u16 1 items=["Entrance", "Exit", "Front", "Side"] ("Mirror Number")
                    w1160 = u16 0 items=["Entrance", "Exit", "Front", "Side"] ("Mirror Number")
                    # "Move Mirrors"
                    n620 = call "JYMirrorMove.vi"("error in (no error)"=w1158, "Mirror Position"="Entrance Mirror", "Mirror Number"=w1160, "RefNum In"=w1156) -> ("error out"=w1155:errorcluster)  [unwired: 6 in, 1 out]
                    n621 = call "JYMirrorMove.vi"("error in (no error)"=w1155, "Mirror Position"="Exit Mirror", "Mirror Number"=w1157, "RefNum In"=w1156) -> ("error out"=w1148:errorcluster, "MonoRefNum Out"=w1149:refnum<k7>)  [unwired: 6 in]
                    n622 = call "JYGetMirrorPos.vi"("error in (no error)"=w1148, "Mirror"=w1150, "Refnum In"=w1149) -> ("error out"=w1153:errorcluster, "Current Mirror Position"=w1147:i32, "Refnum Out"=w1152:refnum<k7>)  [unwired: 1 in]
                    n623 = local write "Entrance Mirror\nPosition"(w1147) -> ()
                    n624 = call "JYGetMirrorPos.vi"("error in (no error)"=w1153, "Mirror"=w1151, "Refnum In"=w1152) -> ("error out"=w1145:errorcluster, "Current Mirror Position"=w1146:i32)  [unwired: 1 in, 1 out]
                    n625 = local write "Exit Mirror\nPosition"(w1146) -> ()
                  }
                  frame #3 {
                    w1163 = u16 0 items=["Front Entrance", "Side Entrance", "Front Exit", "Side Exit", "First Intermediate", "Second Intermediate"] ("Slit")
                    # "Set New Slit Positions"
                    n626 = call "JYSlits.vi"("JYMONOLib.IJYMonoReqd"=w1165, "Slit"=w1163, "error in (no error)"=w1164, "Slit Width"="Target\nFront Entrance") -> ("error out"=w1161:errorcluster)  [unwired: 1 in, 1 out]
                  }
                }
              }
            }
          }
        }
        n627 = local read "Close"() -> (w1103:bool)
      }
    }
  }
  n628 = flat-sequence {
    frame #0 {
      n629 = call <vilib>:"Create Report.vi"("window state (normal)"=T3."no change", "report type"=Report_Type."Excel", "template (empty)"=path "D:/desktop/train/TEST1/Save/516中心波长.xlsx") -> ("report out"=w1172:refnum<class "NI_report.lvclass">, "error out"=w1171:errorcluster)  [unwired: 11 in]
      n630 = call-poly <vilib>:"Excel Get Data.vi"("report in"=w1172, "data type"=string[][] [], "error in (no error)"=w1171) -> ("report out"=w1167:refnum<class "NI_report.lvclass">, "data"=w1175:string[][], "error out"=w1166:errorcluster)  [unwired: 10 in]
      n631 = call-dynamic "Dispose Report.vi"("report in"=w1167, "error in (no error)"=w1166) -> ()  [unwired: 13 in, 1 out]
      n632 = Index Array(array=w1175, index (col)=0 ("禁用的索引 (列)")) -> (element=w1177:string[])  [unwired: 1 in]
      n633 = Fract/Exp String To Number(string=w1177) -> (number=→"波长范围":dbl[])  [unwired: 3 in, 1 out]
    }
  }
